vi "H2O_DIAL_NCAR_4CH_v4.06.vi"() -> ()   [LabVIEW 2012]
uses:
  C:/Users/H2ODial/Desktop/Shared Telescope WV DIAL Code/Libraries and VIs/PowerMeterCommands.dll
  Libraries and VIs/PowerMeterCommands.dll
  <vilib>/DAQmx/write.llb/DAQmx Write (Digital 1D Bool NChan 1Samp 1Line).vi
  <vilib>/DAQmx/miscellaneous.llb/DAQmx Fill In Error Info.vi
  <vilib>/Analysis/baseanly.llb/Mean (DBL).vi
  AMCS_Data.vi
  Libraries and VIs/Scalar_Data.vi
  <vilib>/Analysis/NI_AALBase.lvlib
  Libraries and VIs/Scalar_Data_2.vi
  Libraries and VIs/Scalar_Data_4.vi
  Libraries and VIs/Scalar_Data_3.vi
  Libraries and VIs/CLDevIFace.dll
panel:
  out "AMCS_Profile":i32=8
  out "FileHour":i32=17
  out "L_Count":i32=23
  out "sigma_off_total":dbl[](array[numeric])=[5.235525125067343e-25, 5.206358319245337e-25, 5.177318750524933e-25, 5.148406424862825e-25, 5.119621341127451e-25, 5.090963491196627e-25, 5.062432860011865e-25, 5.034029425635027e-25, 5.005753159352157e-25, 4.977604025706667e-25, 4.949581982592347e-25, 4.921686981325722e-25, 4.893918966711095e-25, 4.866277877122191e-25, 4.8387636445644285e-25, 4.811376194764721e-25, 4.784115447230487e-25, 4.756981315339233e-25, 4.729973706394386e-25, 4.703092521721628e-25, 4.6763376567211625e-25, 4.6497090009594435e-25, 4.623206438225019e-25, 4.596829846622293e-25, 4.57057909862005e-25, 4.544454061150213e-25, 4.518454595652437e-25, 4.492580558158126e-25, 4.4668317993693425e-25, 4.441208164702635e-25, 4.41570949437918e-25, 4.390335623482575e-25, 4.365086382028137e-25, 4.339961595028071e-25, 4.314961082547237e-25, 4.290084659777996e-25, 4.2653321370993085e-25, 4.240703320135042e-25, 4.216198009811418e-25, 4.191816002426457e-25, 4.16755708969195e-25, 4.143421058805604e-25, 4.1194076924960845e-25, 4.095516769084665e-25, 4.0717480625238245e-25, 4.0481013424706545e-25, 4.0245763743206737e-25, 4.001172919260011e-25, 3.977890734322512e-25, 3.9547295724256756e-25, 3.931689182419048e-25, 3.908769309139365e-25, 3.8859696934393876e-25, 3.863290072236815e-25, 3.840730178557474e-25, 3.8182897415734565e-25, 3.7959684866403156e-25, 3.773766135338825e-25, 3.7516824055099053e-25, 3.729717011286995e-25, 3.707869663137923e-25, 3.686140067893342e-25, 3.664527928779591e-25, 3.643032945453827e-25, 3.621654814033011e-25, 3.600393227122229e-25, 3.579247873843723e-25, 3.5582184398664743e-25, 3.5373046074361216e-25, 3.5165060553938904e-25, 3.4958224592064764e-25, 3.475253490990589e-25, 3.454798819536632e-25, 3.4344581103303625e-25, 3.414231025576395e-25, 3.394117224218377e-25, 3.37411636196096e-25, 3.3542280912885406e-25, 3.3344520614845767e-25, 3.3147879186525413e-25, 3.295235305730259e-25, 3.275793862509532e-25, 3.2564632256504646e-25, 3.237243028702917e-25, 3.2181329021119735e-25, 3.1991324732434905e-25, 3.180241366390581e-25, 3.161459202790299e-25, 3.142785600633377e-25, 3.1242201750825597e-25, 3.1057625382770893e-25, 3.0874122993477767e-25, 3.0691690644282785e-25, 3.051032436660927e-25, 3.0330020162078266e-25, 3.0150774002602592e-25, 2.997258183045521e-25, 2.979543955833093e-25, 2.961934306943937e-25, 2.944428821752431e-25, 2.9270270826932477e-25, 2.909728669267514e-25, 2.8925331580414936e-25, 2.875440122654977e-25, 2.8584491338173137e-25, 2.841559759313169e-25, 2.8247715639976386e-25, 2.80808410980223e-25, 2.791496955724979e-25, 2.775009657833479e-25, 2.7586217692567447e-25, 2.742332840183121e-25, 2.7261424178518227e-25, 2.710050046547509e-25, 2.6940552675881075e-25, 2.6781576193155516e-25, 2.6623566370876434e-25, 2.646651853260364e-25, 2.6310427971768174e-25, 2.615528995144771e-25, 2.600109970428841e-25, 2.5847852432207883e-25, 2.569554330624564e-25, 2.554416746633416e-25, 2.5393720020962457e-25, 2.5244196047033826e-25, 2.5095590589459477e-25, 2.4947898660936654e-25, 2.480111524155541e-25, 2.4655235278440513e-25, 2.451025368544176e-25, 2.436616534266772e-25, 2.422296509605852e-25, 2.408064775697375e-25, 2.3939208101763006e-25, 2.3798640871112015e-25, 2.365894076971971e-25, 2.352010246556833e-25, 2.3382120589521406e-25, 2.324498973455175e-25, 2.3108704455300754e-25, 2.2973259267270024e-25, 2.283864864626908e-25, 2.270486702764721e-25, 2.257190880557015e-25, 2.2439768332388837e-25, 2.2308439917739663e-25, 2.2177917827749597e-25, 2.20481962844103e-25, 2.19192694645104e-25, 2.179113149897461e-25, 2.166377647190967e-25, 2.153719841983278e-25, 2.1411391330535246e-25, 2.1286349142540036e-25, 2.1162065743868337e-25, 2.103853497130775e-25, 2.091575060946101e-25, 2.079370638983031e-25, 2.0672395989815037e-25, 2.0551813031976677e-25, 2.0431951082869756e-25, 2.0312803652523447e-25, 2.019436419319984e-25, 2.0076626098781596e-25, 1.9959582703908636e-25, 1.9843227283026113e-25, 1.9727553050009988e-25, 1.9612553156963306e-25, 1.9498220693936616e-25, 1.9384548688025462e-25, 1.9271530103114487e-25, 1.915915783921294e-25, 1.9047424731896738e-25, 1.8936323552292957e-25, 1.8825847006561212e-25, 1.8715987735714719e-25, 1.8606738315918164e-25, 1.8498091257941087e-25, 1.8390039007904753e-25, 1.8282573946936752e-25, 1.8175688392200846e-25, 1.80693745969556e-25, 1.7963624751388698e-25, 1.7858430983630522e-25, 1.7753785360393623e-25, 1.7649679888396773e-25, 1.7546106515613228e-25, 1.7443057132789558e-25, 1.7340523575155863e-25, 1.723849762422857e-25, 1.7136971010131167e-25, 1.7035935413825008e-25, 1.6935382469544605e-25, 1.6835303767796407e-25, 1.6735690858143057e-25, 1.6636535252563445e-25, 1.653782842907513e-25, 1.643956183497921e-25, 1.6341726891478545e-25, 1.624431499756322e-25, 1.6147317534796005e-25, 1.6050725871551994e-25, 1.5954531368896971e-25, 1.585872538492723e-25, 1.576329928151117e-25, 1.566824442883223e-25, 1.5573552212546758e-25, 1.5479214039898043e-25, 1.5385221346219397e-25, 1.5291565602013113e-25, 1.519823831962039e-25, 1.5105231061650234e-25, 1.5012535447460145e-25, 1.49201431624485e-25, 1.482804596459418e-25, 1.4736235693849326e-25, 1.46447042805166e-25, 1.455344375360034e-25, 1.4462446250285657e-25, 1.4371704024629248e-25, 1.4281209456557682e-25, 1.4190955061389853e-25, 1.410093350012645e-25, 1.4011137586880333e-25, 1.3921560301221658e-25, 1.3832194795253431e-25, 1.3743034404767374e-25, 1.3654072658699072e-25, 1.3565303288298996e-25, 1.3476720236918642e-25, 1.3388317669734332e-25, 1.3300089982893968e-25, 1.3212031812258562e-25, 1.3124138043688156e-25, 1.3036403820696332e-25, 1.2948824553577423e-25, 1.2861395928315612e-25, 1.2774113913410786e-25, 1.2686974768684636e-25, 1.2599975053009544e-25, 1.2513111630057894e-25, 1.2426381676023619e-25, 1.2339782685325752e-25, 1.2253312476934588e-25, 1.2166969199403071e-25, 1.2080751335374065e-25, 1.1994657705541538e-25, 1.1908687474046665e-25, 1.182284014933639e-25, 1.1737115587808914e-25, 1.1651513996305814e-25, 1.1566035931942852e-25, 1.1480682304187532e-25, 1.1395454373665928e-25, 1.1310353751750977e-25, 1.1225382399779688e-25, 1.1140542626706877e-25, 1.1055837085176348e-25, 1.097126877076807e-25, 1.0886841014622313e-25, 1.0802557481625692e-25, 1.07184221622742e-25, 1.0634439369229237e-25, 1.0550613727868173e-25, 1.0466950171251473e-25, 1.038345393031225e-25, 1.0300130526116006e-25, 1.0216985760646603e-25, 1.0134025706453978e-25, 1.0051256696943142e-25, 9.968685315566847e-26, 9.886318383691271e-26, 9.804162950309608e-26, 9.722226278487634e-26, 9.640515833439737e-26, 9.559039270504641e-26]
  out "sigma_on_total":dbl[](array[numeric])=[2.3995833041051826e-23, 2.3922427806028756e-23, 2.384791688746997e-23, 2.3772317103212935e-23, 2.3695645459223834e-23, 2.3617919143098038e-23, 2.353915551299477e-23, 2.3459372086545772e-23, 2.3378586534805352e-23, 2.3296816668418693e-23, 2.3214080430222583e-23, 2.3130395885585187e-23, 2.3045781211857275e-23, 2.2960254689709635e-23, 2.2873834692216713e-23, 2.2786539677232958e-23, 2.26983881761429e-23, 2.2609398786386177e-23, 2.2519590159903235e-23, 2.2428980996764618e-23, 2.233759003334336e-23, 2.2245436035687533e-23, 2.215253778837344e-23, 2.2058914088573995e-23, 2.1964583734229998e-23, 2.1869565519300118e-23, 2.1773878221738038e-23, 2.1677540597169405e-23, 2.1580571372247846e-23, 2.1482989233079665e-23, 2.1384812820738464e-23, 2.1286060722317668e-23, 2.11867514639952e-23, 2.108690350380322e-23, 2.0986535223192663e-23, 2.0885664921990106e-23, 2.078431081122936e-23, 2.068249100616584e-23, 2.0580223519476976e-23, 2.0477526256926665e-23, 2.037441700865306e-23, 2.0270913446113544e-23, 2.0167033114661947e-23, 2.0062793429495973e-23, 1.9958211667723764e-23, 1.985330496739564e-23, 1.9748090319499057e-23, 1.9642584563764407e-23, 1.9536804385991807e-23, 1.9430766311537824e-23, 1.9324486701686134e-23, 1.9217981751967428e-23, 1.9111267485338587e-23, 1.9004359749995074e-23, 1.889727421646792e-23, 1.8790026374021327e-23, 1.8682631527238793e-23, 1.8575104794097395e-23, 1.84674611029044e-23, 1.835971518898627e-23, 1.8251881594141955e-23, 1.814397466323634e-23, 1.803600854226578e-23, 1.7927997177436358e-23, 1.781995431311586e-23, 1.7711893489953737e-23, 1.7603828043585478e-23, 1.7495771103906582e-23, 1.7387735594900776e-23, 1.7279734231695694e-23, 1.7171779521110194e-23, 1.7063883761078407e-23, 1.6956059040208986e-23, 1.6848317237070065e-23, 1.6740670020423286e-23, 1.663312884876634e-23, 1.6525704970810114e-23, 1.6418409425264909e-23, 1.6311253041149504e-23, 1.6204246439001306e-23, 1.6097400030205636e-23, 1.5990724018419113e-23, 1.5884228399513838e-23, 1.577792296435066e-23, 1.5671817296197546e-23, 1.5565920775619874e-23, 1.5460242578862832e-23, 1.535479168018885e-23, 1.5249576851998408e-23, 1.514460666843388e-23, 1.5039889504141115e-23, 1.4935433537260487e-23, 1.4831246751329234e-23, 1.472733693540472e-23, 1.4623711686480822e-23, 1.4520378411573963e-23, 1.4417344329131002e-23, 1.431461647050052e-23, 1.4212201682885124e-23, 1.4110106629829185e-23, 1.4008337793905047e-23, 1.3906901479412008e-23, 1.3805803812661607e-23, 1.3705050746147406e-23, 1.360464805856419e-23, 1.3504601358671784e-23, 1.3404916085744038e-23, 1.33055975141312e-23, 1.3206650752755123e-23, 1.3108080749361715e-23, 1.300989229142433e-23, 1.2912090009400432e-23, 1.2814678378339959e-23, 1.2717661720819296e-23, 1.2621044208258517e-23, 1.2524829863555887e-23, 1.2429022564345148e-23, 1.2333626044024168e-23, 1.2238643895015358e-23, 1.2144079569516218e-23, 1.2049936384300202e-23, 1.1956217520538888e-23, 1.1862926027653837e-23, 1.1770064825596866e-23, 1.1677636705336423e-23, 1.1585644333848872e-23, 1.1494090253993612e-23, 1.140297688856002e-23, 1.1312306541333314e-23, 1.1222081399347362e-23, 1.1132303536262725e-23, 1.1042974913417118e-23, 1.095409738203383e-23, 1.0865672685970165e-23, 1.077770246442273e-23, 1.069018825184856e-23, 1.0603131482864411e-23, 1.0516533491872498e-23, 1.0430395517331488e-23, 1.0344718701655819e-23, 1.0259504095410726e-23, 1.0174752657463625e-23, 1.0090465258313015e-23, 1.0006642681274029e-23, 9.92328562444393e-24, 9.840394703656403e-24, 9.757970453103036e-24, 9.676013327237633e-24, 9.594523704137527e-24, 9.513501885337853e-24, 9.432948099139377e-24, 9.352862501650117e-24, 9.273245179271553e-24, 9.194096148754277e-24, 9.115415361305784e-24, 9.037202702127212e-24, 8.95945799326533e-24, 8.882180995005424e-24, 8.805371407477425e-24, 8.729028871786063e-24, 8.653152972477945e-24, 8.577743237723576e-24, 8.502799142614571e-24, 8.428320108863437e-24, 8.354305507372407e-24, 8.280754659437585e-24, 8.207666837515396e-24, 8.135041268097952e-24, 8.062877131154292e-24, 7.99117356294852e-24, 7.919929656301442e-24, 7.84914446290975e-24, 7.778816993979177e-24, 7.708946221065343e-24, 7.639531078293294e-24, 7.570570462739891e-24, 7.50206323561057e-24, 7.434008224352779e-24, 7.366404222220212e-24, 7.299249990914871e-24, 7.232544260133964e-24, 7.166285730139122e-24, 7.100473071653504e-24, 7.035104927252298e-24, 6.970179912711283e-24, 6.905696617243793e-24, 6.841653604993835e-24, 6.778049415778176e-24, 6.71488256599146e-24, 6.652151549491076e-24, 6.5898548382920406e-24, 6.527990883757523e-24, 6.466558117249894e-24, 6.4055549507723266e-24, 6.344979778092631e-24, 6.28483097518053e-24, 6.225106901127807e-24, 6.165805899041039e-24, 6.106926296119407e-24, 6.048466405156796e-24, 5.9904245247443424e-24, 5.932798940248885e-24, 5.875587923847452e-24, 5.81878973608226e-24, 5.762402625414115e-24, 5.7064248300296764e-24, 5.6508545770856186e-24, 5.595690084324867e-24, 5.540929560331407e-24, 5.4865712049292154e-24, 5.432613209855631e-24, 5.379053758857358e-24, 5.325891029033336e-24, 5.273123190347269e-24, 5.220748407202883e-24, 5.1687648376764325e-24, 5.117170634787307e-24, 5.065963946793787e-24, 5.015142917355626e-24, 4.964705686339599e-24, 4.914650389956907e-24, 4.864975161029941e-24, 4.81567812950341e-24, 4.766757423304431e-24, 4.718211167461553e-24, 4.670037486052705e-24, 4.622234501071692e-24, 4.574800333610437e-24, 4.5277331040472795e-24, 4.4810309321178136e-24, 4.4346919373328924e-24, 4.38871423937983e-24, 4.3430959582840964e-24, 4.297835214458712e-24, 4.252930129523995e-24, 4.208378826002288e-24, 4.164179427788139e-24, 4.120330060596267e-24, 4.0768288516550796e-24, 4.033673930358468e-24, 3.990863428575472e-24, 3.9483954803378585e-24, 3.9062682224559106e-24, 3.8644797945055325e-24, 3.823028339213923e-24, 3.781912002534402e-24, 3.741128933721167e-24, 3.700677285403917e-24, 3.660555214319274e-24, 3.620760880699127e-24, 3.581292448804293e-24, 3.5421480872458e-24, 3.5033259686601366e-24, 3.4648242702967565e-24, 3.4266411737802344e-24, 3.3887748653248774e-24, 3.35122353602395e-24, 3.313985381867669e-24, 3.2770586035106233e-24, 3.2404414071352855e-24, 3.2041320036199322e-24, 3.168128609466342e-24, 3.1324294461445785e-24, 3.097032740909227e-24, 3.061936726152549e-24, 3.0271396401184125e-24, 2.9926397264979493e-24, 2.958435234734132e-24, 2.9245244200823504e-24, 2.8909055435197247e-24, 2.857576871953275e-24, 2.8245366782699725e-24, 2.7917832411696796e-24, 2.7593148455736252e-24, 2.727129782308357e-24, 2.6952263482932426e-24, 2.663602846782851e-24]
  out "background start":u32=269
  in  "Tab Control 2":enum32{"WV ND far", "WV ND near"}(tab)
  out "Water Vapor Number Density":dbl[][](graph)=[[-1.2429232877484484, -0.1516675083101968, -0.2538905255591858, -0.8248790705144008, -0.7242099736682136, -0.00381566942216356, 0.5865003613322888, 0.8338027871213243, 0.9701605815337504, 1.1834523029548778, 1.5190287098751127, 1.7810431574320749, 1.6746765343626566, 1.1151725227331368, 0.46655235793116506, 0.35715468660627175, 0.6669999198229103, 0.6229583187384804, 0.5589044475896486, 0.7015386580818149, 0.4798277530250588, 0.5321622767939538, 0.7626570360936702, 0.548610948648949, 0.9084936586508549, 1.2026792009723286, 0.774704699408754, 0.5215060631479779, 0.12261891062905873, 0.21928947886161568, 0.8338105270444128, 0.7207357046057596, 0.7010869622309128, 1.3141939911674185, 0.9797233881152331, 0.17444693844264145, 0.8196905370743147, 1.2982930105898909, 0.11109624339884688, -0.43162778210005126, 0.5989210399599628, 0.8290997131095186, 0.9085277187984653, 1.1666295347768159, 1.4953864166373505, 0.973830244036953, 0.40024763155462806, 0.40566207310085767, 0.12859842661309212, 0.816329506196804, 1.6877091211861164, 1.4740247437794118, 0.5494960806690096, 0.14364505636130315, 1.6910867165083499, 2.541349269410972, 3.0215147517757615, 5.116023264360957, 11.66361642135062, 15.732511596518307, 11.746439379020979, 10.179584454030591, 9.832529406708609, 8.268647831389469, 4.724342168222102, -5.092206912585782, -13.3625201348692, -20.76218607865762, -31.481285721313007, -38.11141827571821, -31.134574912835927, -23.05395421124333, -18.75920646807871, -11.6291784332, -9.182440744289961, 3.6065364004744884, 14.28272592509906, 16.011915781887442, 21.469311288754138, 22.06574013828088, 12.21267680703055, 7.045281295181791, 5.126441440726531, 2.1140699610393394, 4.549659394917577, 5.4053975728869545, -1.494856115972021, -1.1471850648222977, -2.2964282267520684, -1.701978840115399, 6.926942778338519, -5.157508026215396, -16.63199538963445, -9.965627988382359, -9.996745428358686, -11.837454532000542, -7.791885667567633, -8.680656157447176, -8.91275723505151, -1.6980976668310848, -2.133416024855749, 6.9027910551985565, 15.630215820196536, 9.119408516902418, 13.419777247258404, 3.714772754413472, -1.0207358839785408, 1.9570108859042183, 8.45768550919551, 5.500832494929015, 9.619107112547066, 3.5429906655082815, 2.281420809371128, 3.3348498361329115, 13.33869517507839, 20.282683395031995, 12.958395546058279, 12.790251903025284, 5.239171426669377, 5.18576865128037, -7.793357814133322, -4.368293566880555, -3.168338430754624, -3.568868023379041, -19.349826708428175, -18.20847151281235, -6.272910319204182, -5.810405292731198, 0.03778017829370816, 1.6447693871034739, 12.138812274569242, 22.264002949155152, 20.98736700005724, 5.225366734954423, -4.2130058766847345, -5.530836082222857, -7.678583545699047, 2.8238125624467885, 4.404424187372618, -16.837237405438508, -25.11428016723591, -32.56648715841542, -51.93781123610291, -12.449234368136176, -7.120712329696384, -7.810751630429527, -5.682295948947324, -14.881668117301965, -17.89571509714611, 21.5597299249097, 14.887365183365386, 9.094029084786875, 39.765998068462736, 26.698821470330174, 5.3888067881035235, 36.31266939640943, 23.52473002015805, 7.885320353358003, 4.491673034757693, -25.66484118463619, -24.784846332156523, -11.314522471658744, -8.629722713276472, -36.47960588329874, 3.344643837569838, -43.4685580824685, -21.017479049621816, -13.573236011339208, 1.4056605605320718, 20.621744510192077, 48.534446642723786, 18.043662576249712, 18.729984852689935, 15.453816513065464, -16.562572588412568, -1.75727853159035, 12.077447417423167, 23.28859626581528, 8.189331760622546, -10.325523115047803, -24.985943747309573, 11.02611193863362, -21.194886596636273, -3.3737336795583666, 12.356163073717218, 19.49913906422601, -31.903517194256743, -28.34741638064177, -22.84649773688388, -3.7322150184329868, -7.133598473140854, -30.506891256676347, 0.8094334644236778, -10.185875717445333, -1.7805612059650464, -18.920780567052645, 18.561020494796015, 32.740090001051776, -10.431965025082278, 24.148735007779216, -12.811558818079975, 22.77751095878245, 3.073515709862989, -1.5964031788087782, 23.237423290854288, -10.171927114726072, -18.071924640995153, -22.573720000403977, 31.51068338334455, -25.15388772107271, -10.403629581588998, -23.273123302299926, -0.7696347470225127, 28.138111524189863, -53.130668832773836, 19.25820068507475, 30.433478138971022, 4.601226158871911, -7.687709637981916, 26.504732966928117, -6.453108031183767, 12.133560044433468, -17.91335412457681, -27.611164781409965, 58.267542043909756, 27.655747672019785, 10.074228863403778, -15.797465265403272, 29.104671664483025, -20.527102926569924, 71.93119794505054, 8.975498249493553, -3.3375393334362444, 25.152309034601856, -9.70197245913663, -28.78587032628703, -37.26876049881305, -21.358169118247066, -42.25654771519554, 38.05236561426804, -21.06199519179915, -19.681897042577624, -33.54178592739098, -8.38025346936163, -9.769431139416938, 11.584675554539887, 6.052684205738731, 15.000220216910806, -37.12617526141696, -19.779582424384554, 7.072374690381783, 9.593917717650474, 9.722908351927563, -19.755356323145175, 1.5520809859448423, 32.36319254600239, 31.348864192718274, -34.65191626742631, 18.898751794149703, -13.173451913530773, -79.37971946570717, -82.26941833977881, 51.361564922853184, 37.72821751239603, 23.664211401877278, -159.38500039414865, 63.63015044438198, 87.46258784324492, 124.20770000486162, 110.10692816340169, 58.297939579874345, 90.76767995026964, -0.5951627932311193, -15.350600261615488, -23.944134589509243, 130.0552581066162, 0.0, 0.0, 0.0, 0.0]]
  out "Water Vapor Number Density 2":dbl[][](graph)=[[nan, nan, nan, nan, nan, nan, nan, nan, nan, nan, nan, nan, nan, nan, nan, nan, nan, nan, nan, nan, nan, nan, nan, nan, nan, nan, nan, nan, nan, nan, nan, nan, nan, nan, nan, nan, nan, nan, nan, nan, nan, nan, nan, nan, nan, nan, nan, nan, nan, nan, nan, nan, nan, nan, nan, nan, nan, nan, nan, nan, nan, nan, nan, nan, nan, nan, nan, nan, nan, nan, nan, nan, nan, nan, nan, nan, nan, nan, nan, nan, nan, nan, nan, nan, nan, nan, nan, nan, nan, nan, nan, nan, nan, nan, nan, nan, nan, nan, nan, nan, nan, nan, nan, nan, nan, nan, nan, nan, nan, nan, nan, nan, nan, nan, nan, nan, nan, nan, nan, nan, nan, nan, nan, nan, nan, nan, nan, nan, nan, nan, nan, nan, nan, nan, nan, nan, nan, nan, nan, nan, nan, nan, nan, nan, nan, nan, nan, nan, nan, nan, nan, nan, nan, nan, nan, nan, nan, nan, nan, nan, nan, nan, nan, nan, nan, nan, nan, nan, nan, nan, nan, nan, nan, nan, nan, nan, nan, nan, nan, nan, nan, nan, nan, nan, nan, nan, nan, nan, nan, nan, nan, nan, nan, nan, nan, nan, nan, nan, nan, nan, nan, nan, nan, nan, nan, nan, nan, nan, nan, nan, nan, nan, nan, nan, nan, nan, nan, nan, nan, nan, nan, nan, nan, nan, nan, nan, nan, nan, nan, nan, nan, nan, nan, nan, nan, nan, nan, nan, nan, nan, nan, nan, nan, nan, nan, nan, nan, nan, nan, nan, nan, nan, nan, nan, nan, nan, nan, nan, nan, nan, nan, nan, nan, nan, nan, nan, nan, nan, nan, nan, nan, nan, nan, nan, nan, nan, 0.0, 0.0, 0.0, 0.0]] caption="Water Vapor Number Density"
  out "RingBuffer offline near":dbl[][](array[numeric])
  out "RingBuffer aerosol near":dbl[][](array[numeric])
  in  "?":T1(tab)=enum."Raw Counts far"
  out "NRB":dbl[][](graph)=[[nan, nan, nan, nan, nan, nan, nan, nan, nan, nan, nan, nan, nan, nan, nan, nan, nan, nan, nan, nan, nan, nan, nan, nan, nan, nan, nan, nan, nan, nan, nan, nan, nan, nan, nan, nan, nan, nan, nan, nan, nan, nan, nan, nan, nan, nan, nan, nan, nan, nan, nan, nan, nan, nan, nan, nan, nan, nan, nan, nan, nan, nan, nan, nan, nan, nan, nan, nan, nan, nan, nan, nan, nan, nan, nan, nan, nan, nan, nan, nan, nan, nan, nan, nan, nan, nan, nan, nan, nan, nan, nan, nan, nan, nan, nan, nan, nan, nan, nan, nan, nan, nan, nan, nan, nan, nan, nan, nan, nan, nan, nan, nan, nan, nan, nan, nan, nan, nan, nan, nan, nan, nan, nan, nan, nan, nan, nan, nan, nan, nan, nan, nan, nan, nan, nan, nan, nan, nan, nan, nan, nan, nan, nan, nan, nan, nan, nan, nan, nan, nan, nan, nan, nan, nan, nan, nan, nan, nan, nan, nan, nan, nan, nan, nan, nan, nan, nan, nan, nan, nan, nan, nan, nan, nan, nan, nan, nan, nan, nan, nan, nan, nan, nan, nan, nan, nan, nan, nan, nan, nan, nan, nan, nan, nan, nan, nan, nan, nan, nan, nan, nan, nan, nan, nan, nan, nan, nan, nan, nan, nan, nan, nan, nan, nan, nan, nan, nan, nan, nan, nan, nan, nan, nan, nan, nan, nan, nan, nan, nan, nan, nan, nan, nan, nan, nan, nan, nan, nan, nan, nan, nan, nan, nan, nan, nan, nan, nan, nan, nan, nan, nan, nan, nan, nan, nan, nan, nan, nan, nan, nan, nan, nan, nan, nan, nan, nan, nan, nan, nan, nan, nan, nan, nan, nan, nan, nan, nan, 0.0, 0.0, 0.0]] caption="Water Vapor Number Density"
  out "NRB 2":dbl[][](graph)=[[nan, nan, nan, nan, nan, nan, nan, nan, nan, nan, nan, nan, nan, nan, nan, nan, nan, nan, nan, nan, nan, nan, nan, nan, nan, nan, nan, nan, nan, nan, nan, nan, nan, nan, nan, nan, nan, nan, nan, nan, nan, nan, nan, nan, nan, nan, nan, nan, nan, nan, nan, nan, nan, nan, nan, nan, nan, nan, nan, nan, nan, nan, nan, nan, nan, nan, nan, nan, nan, nan, nan, nan, nan, nan, nan, nan, nan, nan, nan, nan, nan, nan, nan, nan, nan, nan, nan, nan, nan, nan, nan, nan, nan, nan, nan, nan, nan, nan, nan, nan, nan, nan, nan, nan, nan, nan, nan, nan, nan, nan, nan, nan, nan, nan, nan, nan, nan, nan, nan, nan, nan, nan, nan, nan, nan, nan, nan, nan, nan, nan, nan, nan, nan, nan, nan, nan, nan, nan, nan, nan, nan, nan, nan, nan, nan, nan, nan, nan, nan, nan, nan, nan, nan, nan, nan, nan, nan, nan, nan, nan, nan, nan, nan, nan, nan, nan, nan, nan, nan, nan, nan, nan, nan, nan, nan, nan, nan, nan, nan, nan, nan, nan, nan, nan, nan, nan, nan, nan, nan, nan, nan, nan, nan, nan, nan, nan, nan, nan, nan, nan, nan, nan, nan, nan, nan, nan, nan, nan, nan, nan, nan, nan, nan, nan, nan, nan, nan, nan, nan, nan, nan, nan, nan, nan, nan, nan, nan, nan, nan, nan, nan, nan, nan, nan, nan, nan, nan, nan, nan, nan, nan, nan, nan, nan, nan, nan, nan, nan, nan, nan, nan, nan, nan, nan, nan, nan, nan, nan, nan, nan, nan, nan, nan, nan, nan, nan, nan, nan, nan, nan, nan, nan, nan, nan, nan, nan, nan, 0.0, 0.0, 0.0]] caption="Water Vapor Number Density"
  out "raw counts":dbl[][](graph) caption="Water Vapor Number Density"
  out "raw counts near":dbl[][](graph) caption="Water Vapor Number Density"
  out "Aerosol Smoothed 2":dbl[](array[numeric])
  out "Off-Line Smoothed 2":dbl[](array[numeric])
  out "Off-Line Bin Readings 2":dbl[](array[numeric])
  out "On-Line Smoothed 2":dbl[](array[numeric])
  out "On-Line Bin Readings 2":dbl[](array[numeric])
  in  "stop":bool
  in  "Reset Average":bool=TRUE
  in  "Save Data?":bool=TRUE
  in  "Collect Data?":bool=TRUE
  in  "ILX Address":i32=6 min=0 step=1
  in  "Lambda On DBR Current":dbl=170.37999999999937
  in  "Lambda Off DBR Current":dbl=172.63
  in  "Tab Control":T2(tab)=enum."g/m^3"
  out "Water Vapor Number Density  2":cluster{"Y":dbl[], "Y":dbl[]}[](graph)=[{"Y"=array[276 elements], "Y"=array[280 elements]}, {"Y"=[nan, nan, nan, nan, nan, nan, nan, nan, nan, nan, nan, nan, nan, nan, nan, nan, nan, nan, nan, nan, nan, nan, nan, nan, nan, nan, nan, nan, nan, nan, nan, nan, nan, nan, nan, nan, nan, nan, nan, nan, nan, nan, nan, nan, nan, nan, nan, nan, nan, nan, nan, nan, nan, nan, nan, nan, nan, nan, nan, nan, nan, nan, nan, nan, nan, nan, nan, nan, nan, nan, nan, nan, nan, nan, nan, nan, nan, nan, nan, nan, nan, nan, nan, nan, nan, nan, nan, nan, nan, nan, nan, nan, nan, nan, nan, nan, nan, nan, nan, nan, nan, nan, nan, nan, nan, nan, nan, nan, nan, nan, nan, nan, nan, nan, nan, nan, nan, nan, nan, nan, nan, nan, nan, nan, nan, nan, nan, nan, nan, nan, nan, nan, nan, nan, nan, nan, nan, nan, nan, nan, nan, nan, nan, nan, nan, nan, nan, nan, nan, nan, nan, nan, nan, nan, nan, nan, nan, nan, nan, nan, nan, nan, nan, nan, nan, nan, nan, nan, nan, nan, nan, nan, nan, nan, nan, nan, nan, nan, nan, nan, nan, nan, nan, nan, nan, nan, nan, nan, nan, nan, nan, nan, nan, nan, nan, nan, nan, nan, nan, nan, nan, nan, nan, nan, nan, nan, nan, nan, nan, nan, nan, nan, nan, nan, nan, nan, nan, nan, nan, nan, nan, nan, nan, nan, nan, nan, nan, nan, nan, nan, nan, nan, nan, nan, nan, nan, nan, nan, nan, nan, nan, nan, nan, nan, nan, nan, nan, nan, nan, nan, nan, nan, nan, nan, nan, nan, nan, nan, nan, nan, nan, nan, nan, nan, nan, nan, nan, nan, nan, nan, nan, nan, nan, nan, nan, nan], "Y"=array[280 elements]}]
  out "Absolute Humidity":cluster{"Y":dbl[], "Y":dbl[]}[](graph)=[{"Y"=array[276 elements], "Y"=array[280 elements]}, {"Y"=[nan, nan, nan, nan, nan, nan, nan, nan, nan, nan, nan, nan, nan, nan, nan, nan, nan, nan, nan, nan, nan, nan, nan, nan, nan, nan, nan, nan, nan, nan, nan, nan, nan, nan, nan, nan, nan, nan, nan, nan, nan, nan, nan, nan, nan, nan, nan, nan, nan, nan, nan, nan, nan, nan, nan, nan, nan, nan, nan, nan, nan, nan, nan, nan, nan, nan, nan, nan, nan, nan, nan, nan, nan, nan, nan, nan, nan, nan, nan, nan, nan, nan, nan, nan, nan, nan, nan, nan, nan, nan, nan, nan, nan, nan, nan, nan, nan, nan, nan, nan, nan, nan, nan, nan, nan, nan, nan, nan, nan, nan, nan, nan, nan, nan, nan, nan, nan, nan, nan, nan, nan, nan, nan, nan, nan, nan, nan, nan, nan, nan, nan, nan, nan, nan, nan, nan, nan, nan, nan, nan, nan, nan, nan, nan, nan, nan, nan, nan, nan, nan, nan, nan, nan, nan, nan, nan, nan, nan, nan, nan, nan, nan, nan, nan, nan, nan, nan, nan, nan, nan, nan, nan, nan, nan, nan, nan, nan, nan, nan, nan, nan, nan, nan, nan, nan, nan, nan, nan, nan, nan, nan, nan, nan, nan, nan, nan, nan, nan, nan, nan, nan, nan, nan, nan, nan, nan, nan, nan, nan, nan, nan, nan, nan, nan, nan, nan, nan, nan, nan, nan, nan, nan, nan, nan, nan, nan, nan, nan, nan, nan, nan, nan, nan, nan, nan, nan, nan, nan, nan, nan, nan, nan, nan, nan, nan, nan, nan, nan, nan, nan, nan, nan, nan, nan, nan, nan, nan, nan, nan, nan, nan, nan, nan, nan, nan, nan, nan, nan, nan, nan, nan, nan, nan, nan, nan, nan], "Y"=array[280 elements]}]
  out "NRB plot":cluster{"Y":dbl[], "Y":dbl[]}[](graph)=[{"Y"=[nan, nan, nan, nan, nan, nan, nan, nan, nan, nan, nan, nan, nan, nan, nan, nan, nan, nan, nan, nan, nan, nan, nan, nan, nan, nan, nan, nan, nan, nan, nan, nan, nan, nan, nan, nan, nan, nan, nan, nan, nan, nan, nan, nan, nan, nan, nan, nan, nan, nan, nan, nan, nan, nan, nan, nan, nan, nan, nan, nan, nan, nan, nan, nan, nan, nan, nan, nan, nan, nan, nan, nan, nan, nan, nan, nan, nan, nan, nan, nan, nan, nan, nan, nan, nan, nan, nan, nan, nan, nan, nan, nan, nan, nan, nan, nan, nan, nan, nan, nan, nan, nan, nan, nan, nan, nan, nan, nan, nan, nan, nan, nan, nan, nan, nan, nan, nan, nan, nan, nan, nan, nan, nan, nan, nan, nan, nan, nan, nan, nan, nan, nan, nan, nan, nan, nan, nan, nan, nan, nan, nan, nan, nan, nan, nan, nan, nan, nan, nan, nan, nan, nan, nan, nan, nan, nan, nan, nan, nan, nan, nan, nan, nan, nan, nan, nan, nan, nan, nan, nan, nan, nan, nan, nan, nan, nan, nan, nan, nan, nan, nan, nan, nan, nan, nan, nan, nan, nan, nan, nan, nan, nan, nan, nan, nan, nan, nan, nan, nan, nan, nan, nan, nan, nan, nan, nan, nan, nan, nan, nan, nan, nan, nan, nan, nan, nan, nan, nan, nan, nan, nan, nan, nan, nan, nan, nan, nan, nan, nan, nan, nan, nan, nan, nan, nan, nan, nan, nan, nan, nan, nan, nan, nan, nan, nan, nan, nan, nan, nan, nan, nan, nan, nan, nan, nan, nan, nan, nan, nan, nan, nan, nan, nan, nan, nan, nan, nan, nan, nan, nan, nan, nan, nan, nan, nan, nan, nan], "Y"=[0.075, 0.15, 0.22499999999999998, 0.3, 0.375, 0.45, 0.5249999999999999, 0.6, 0.6749999999999999, 0.7499999999999999, 0.825, 0.8999999999999999, 0.9749999999999999, 1.05, 1.125, 1.2, 1.275, 1.3499999999999999, 1.4249999999999998, 1.5, 1.575, 1.65, 1.7249999999999999, 1.7999999999999998, 1.8749999999999998, 1.95, 2.025, 2.1, 2.1750000000000003, 2.25, 2.325, 2.4, 2.475, 2.5500000000000003, 2.625, 2.7, 2.775, 2.85, 2.9250000000000003, 3.0, 3.075, 3.15, 3.225, 3.3000000000000003, 3.375, 3.45, 3.525, 3.6, 3.675, 3.75, 3.825, 3.9, 3.975, 4.05, 4.125, 4.2, 4.275, 4.35, 4.425, 4.5, 4.575, 4.65, 4.725, 4.8, 4.875, 4.95, 5.025, 5.1, 5.175, 5.25, 5.325, 5.4, 5.475, 5.55, 5.625, 5.7, 5.775, 5.85, 5.925, 6.0, 6.075, 6.15, 6.225, 6.3, 6.375, 6.45, 6.525, 6.6, 6.675, 6.75, 6.825, 6.9, 6.975, 7.05, 7.125, 7.2, 7.2749999999999995, 7.35, 7.425, 7.5, 7.575, 7.6499999999999995, 7.725, 7.8, 7.875, 7.95, 8.024999999999999, 8.1, 8.174999999999999, 8.249999999999998, 8.325, 8.399999999999999, 8.475, 8.549999999999999, 8.624999999999998, 8.7, 8.774999999999999, 8.85, 8.924999999999999, 8.999999999999998, 9.075, 9.149999999999999, 9.225, 9.299999999999999, 9.374999999999998, 9.45, 9.524999999999999, 9.6, 9.674999999999999, 9.749999999999998, 9.825, 9.899999999999999, 9.975, 10.049999999999999, 10.124999999999998, 10.2, 10.274999999999999, 10.35, 10.424999999999999, 10.499999999999998, 10.575, 10.649999999999999, 10.725, 10.799999999999999, 10.874999999999998, 10.95, 11.024999999999999, 11.1, 11.174999999999999, 11.249999999999998, 11.325, 11.399999999999999, 11.475, 11.549999999999999, 11.624999999999998, 11.7, 11.774999999999999, 11.85, 11.924999999999999, 11.999999999999998, 12.075, 12.149999999999999, 12.225, 12.299999999999999, 12.374999999999998, 12.45, 12.524999999999999, 12.6, 12.674999999999999, 12.749999999999998, 12.825, 12.899999999999999, 12.975, 13.049999999999999, 13.124999999999998, 13.2, 13.274999999999999, 13.35, 13.424999999999999, 13.499999999999998, 13.575, 13.649999999999999, 13.725, 13.799999999999999, 13.874999999999998, 13.95, 14.024999999999999, 14.1, 14.174999999999999, 14.249999999999998, 14.325, 14.399999999999999, 14.474999999999998, 14.549999999999999, 14.624999999999998, 14.7, 14.774999999999999, 14.849999999999998, 14.924999999999999, 14.999999999999998, 15.075, 15.149999999999999, 15.224999999999998, 15.299999999999999, 15.374999999999998, 15.45, 15.524999999999999, 15.599999999999998, 15.674999999999999, 15.749999999999998, 15.825, 15.899999999999999, 15.974999999999998, 16.05, 16.125, 16.2, 16.275, 16.349999999999998, 16.424999999999997, 16.5, 16.575, 16.65, 16.724999999999998, 16.799999999999997, 16.875, 16.95, 17.025, 17.099999999999998, 17.174999999999997, 17.25, 17.325, 17.4, 17.474999999999998, 17.549999999999997, 17.625, 17.7, 17.775, 17.849999999999998, 17.924999999999997, 18.0, 18.075, 18.15, 18.224999999999998, 18.299999999999997, 18.375, 18.45, 18.525, 18.599999999999998, 18.674999999999997, 18.75, 18.825, 18.9, 18.974999999999998, 19.049999999999997, 19.125, 19.2, 19.275, 19.349999999999998, 19.424999999999997, 19.5, 19.575, 19.65, 19.724999999999998, 19.799999999999997, 19.875, 19.95, 20.025, 20.099999999999998, 20.174999999999997, 20.25, 20.325, 20.4, 20.474999999999998, 20.549999999999997, 20.625, 20.7, 20.775, 20.849999999999998, 20.924999999999997, 21.0]}, ...(2 in all)]
  in  "background length":i32=10
  out "Correction":cluster{"Y":dbl[], "Y":dbl[]}[](graph)=[{"Y"=[nan, nan, nan, nan, nan, nan, nan, nan, nan, nan, nan, nan, nan, nan, nan, nan, nan, nan, nan, nan, nan, nan, nan, nan, nan, nan, nan, nan, nan, nan, nan, nan, nan, nan, nan, nan, nan, nan, nan, nan, nan, nan, nan, nan, nan, nan, nan, nan, nan, nan, nan, nan, nan, nan, nan, nan, nan, nan, nan, nan, nan, nan, nan, nan, nan, nan, nan, nan, nan, nan, nan, nan, nan, nan, nan, nan, nan, nan, nan, nan, nan, nan, nan, nan, nan, nan, nan, nan, nan, nan, nan, nan, nan, nan, nan, nan, nan, nan, nan, nan, nan, nan, nan, nan, nan, nan, nan, nan, nan, nan, nan, nan, nan, nan, nan, nan, nan, nan, nan, nan, nan, nan, nan, nan, nan, nan, nan, nan, nan, nan, nan, nan, nan, nan, nan, nan, nan, nan, nan, nan, nan, nan, nan, nan, nan, nan, nan, nan, nan, nan, nan, nan, nan, nan, nan, nan, nan, nan, nan, nan, nan, nan, nan, nan, nan, nan, nan, nan, nan, nan, nan, nan, nan, nan, nan, nan, nan, nan, nan, nan, nan, nan, nan, nan, nan, nan, nan, nan, nan, nan, nan, nan, nan, nan, nan, nan, nan, nan, nan, nan, nan, nan, nan, nan, nan, nan, nan, nan, nan, nan, nan, nan, nan, nan, nan, nan, nan, nan, nan, nan, nan, nan, nan, nan, nan, nan, nan, nan, nan, nan, nan, nan, nan, nan, nan, nan, nan, nan, nan, nan, nan, nan, nan, nan, nan, nan, nan, nan, nan, nan, nan, nan, nan, nan, nan, nan, nan, nan, nan, nan, nan, nan, nan, nan, nan, nan, nan, nan, nan, nan, nan, nan, nan, nan, nan, nan, nan], "Y"=[0.075, 0.15, 0.22499999999999998, 0.3, 0.375, 0.45, 0.5249999999999999, 0.6, 0.6749999999999999, 0.7499999999999999, 0.825, 0.8999999999999999, 0.9749999999999999, 1.05, 1.125, 1.2, 1.275, 1.3499999999999999, 1.4249999999999998, 1.5, 1.575, 1.65, 1.7249999999999999, 1.7999999999999998, 1.8749999999999998, 1.95, 2.025, 2.1, 2.1750000000000003, 2.25, 2.325, 2.4, 2.475, 2.5500000000000003, 2.625, 2.7, 2.775, 2.85, 2.9250000000000003, 3.0, 3.075, 3.15, 3.225, 3.3000000000000003, 3.375, 3.45, 3.525, 3.6, 3.675, 3.75, 3.825, 3.9, 3.975, 4.05, 4.125, 4.2, 4.275, 4.35, 4.425, 4.5, 4.575, 4.65, 4.725, 4.8, 4.875, 4.95, 5.025, 5.1, 5.175, 5.25, 5.325, 5.4, 5.475, 5.55, 5.625, 5.7, 5.775, 5.85, 5.925, 6.0, 6.075, 6.15, 6.225, 6.3, 6.375, 6.45, 6.525, 6.6, 6.675, 6.75, 6.825, 6.9, 6.975, 7.05, 7.125, 7.2, 7.2749999999999995, 7.35, 7.425, 7.5, 7.575, 7.6499999999999995, 7.725, 7.8, 7.875, 7.95, 8.024999999999999, 8.1, 8.174999999999999, 8.249999999999998, 8.325, 8.399999999999999, 8.475, 8.549999999999999, 8.624999999999998, 8.7, 8.774999999999999, 8.85, 8.924999999999999, 8.999999999999998, 9.075, 9.149999999999999, 9.225, 9.299999999999999, 9.374999999999998, 9.45, 9.524999999999999, 9.6, 9.674999999999999, 9.749999999999998, 9.825, 9.899999999999999, 9.975, 10.049999999999999, 10.124999999999998, 10.2, 10.274999999999999, 10.35, 10.424999999999999, 10.499999999999998, 10.575, 10.649999999999999, 10.725, 10.799999999999999, 10.874999999999998, 10.95, 11.024999999999999, 11.1, 11.174999999999999, 11.249999999999998, 11.325, 11.399999999999999, 11.475, 11.549999999999999, 11.624999999999998, 11.7, 11.774999999999999, 11.85, 11.924999999999999, 11.999999999999998, 12.075, 12.149999999999999, 12.225, 12.299999999999999, 12.374999999999998, 12.45, 12.524999999999999, 12.6, 12.674999999999999, 12.749999999999998, 12.825, 12.899999999999999, 12.975, 13.049999999999999, 13.124999999999998, 13.2, 13.274999999999999, 13.35, 13.424999999999999, 13.499999999999998, 13.575, 13.649999999999999, 13.725, 13.799999999999999, 13.874999999999998, 13.95, 14.024999999999999, 14.1, 14.174999999999999, 14.249999999999998, 14.325, 14.399999999999999, 14.474999999999998, 14.549999999999999, 14.624999999999998, 14.7, 14.774999999999999, 14.849999999999998, 14.924999999999999, 14.999999999999998, 15.075, 15.149999999999999, 15.224999999999998, 15.299999999999999, 15.374999999999998, 15.45, 15.524999999999999, 15.599999999999998, 15.674999999999999, 15.749999999999998, 15.825, 15.899999999999999, 15.974999999999998, 16.05, 16.125, 16.2, 16.275, 16.349999999999998, 16.424999999999997, 16.5, 16.575, 16.65, 16.724999999999998, 16.799999999999997, 16.875, 16.95, 17.025, 17.099999999999998, 17.174999999999997, 17.25, 17.325, 17.4, 17.474999999999998, 17.549999999999997, 17.625, 17.7, 17.775, 17.849999999999998, 17.924999999999997, 18.0, 18.075, 18.15, 18.224999999999998, 18.299999999999997, 18.375, 18.45, 18.525, 18.599999999999998, 18.674999999999997, 18.75, 18.825, 18.9, 18.974999999999998, 19.049999999999997, 19.125, 19.2, 19.275, 19.349999999999998, 19.424999999999997, 19.5, 19.575, 19.65, 19.724999999999998, 19.799999999999997, 19.875, 19.95, 20.025, 20.099999999999998, 20.174999999999997, 20.25, 20.325, 20.4, 20.474999999999998, 20.549999999999997, 20.625, 20.7, 20.775, 20.849999999999998, 20.924999999999997, 21.0]}, ...(2 in all)]
  in  "dead time":dbl=3.7e-08
  out "Optical Depth":cluster{"Y":dbl[], "Y":dbl[]}[](graph) caption="XY Graph"
  out "RingBuffer offline far":dbl[][](array[numeric])
  out "RingBuffer aerosol far":dbl[][](array[numeric])
  in  "Weather":T3(tab)=enum."Pulse Energy (Micro Joule)"
  in  "Temperature (C)":dbl=15.0
  out "Temperature (C)":dbl(graph)=15.0
  in  "Pressure (mbar or hPa)":dbl=832.0
  out "Pressure (mb)":dbl(graph)=832.0
  out "Relative Humdity (%)":dbl(graph)=40.0
  out "Pulse Energy (Micro Joule)":T4(graph)={"Online Pulse Energy"=4.73832, "Pulse Energy Offline"=4.74074}
  out "?":cluster{"mean":dbl, "mean":dbl}(graph)={"mean"=nan, "mean"=nan}
  out "Index":i32=24
  out "Aerosol Smoothed":dbl[](array[numeric])=[729.1169811320754, 948.0320754716977, 1131.3245283018864, 1271.796226415094, 1331.5981132075472, 1313.6358490566035, 1265.418867924528, 1198.6924528301884, 1107.6830188679241, 1013.7018867924523, 927.6169811320751, 845.9471698113205, 778.2867924528299, 715.8622641509432, 646.4188679245282, 587.7962264150942, 533.5981132075472, 490.6924528301886, 456.9283018867924, 417.2113207547169, 386.4849056603773, 360.3716981132075, 330.45660377358496, 308.0886792452831, 283.9377358490567, 262.0886792452832, 250.83396226415107, 240.6547169811322, 222.27735849056614, 199.38113207547175, 186.7773584905661, 180.61698113207552, 163.4849056603774, 151.02264150943398, 151.63584905660377, 145.29622641509434, 133.6075471698113, 125.33396226415094, 118.55094339622642, 110.06981132075471, 100.8811320754717, 92.94716981132075, 88.70188679245283, 84.74905660377357, 81.54150943396225, 78.28679245283016, 73.92830188679241, 69.48490566037734, 66.83396226415093, 62.95660377358488, 57.654716981132054, 53.81509433962262, 49.50377358490564, 44.447169811320734, 38.34339622641509, 32.843396226415095, 32.62641509433962, 31.409433962264146, 28.73962264150943, 29.82452830188679, 30.29622641509434, 25.994339622641505, 24.71132075471698, 24.645283018867925, 35.116981132075466, 96.0132075471698, 260.5226415094339, 449.29622641509434, 510.8716981132075, 479.86226415094336, 447.60754716981126, 405.4, 300.45660377358496, 150.04150943396232, 45.09811320754716, 14.17358490566038, 12.881132075471701, 12.75849056603774, 9.805660377358492, 5.843396226415094, 3.9660377358490564, 6.569811320754717, 6.541509433962264, 4.362264150943396, 5.003773584905661, 6.29622641509434, 4.749056603773584, 4.333962264150943, 7.522641509433962, 6.2679245283018865, 3.3716981132075468, 3.6641509433962263, 2.6735849056603773, 5.8339622641509425, 8.192452830188678, 4.758490566037736, 3.843396226415094, 3.5886792452830187, 3.0698113207547166, 3.9660377358490564, 5.409433962264151, 6.1169811320754715, 3.749056603773585, 2.6075471698113204, 2.984905660377358, 1.7773584905660376, 2.9377358490566037, 4.1830188679245275, 5.20188679245283, 3.739622641509434, 2.6358490566037736, 5.135849056603773, 5.569811320754717, 3.7962264150943392, 5.475471698113208, 7.749056603773585, 8.277358490566037, 5.437735849056604, 4.088679245283019, 8.909433962264153, 27.239622641509428, 62.541509433962254, 71.92830188679244, 40.267924528301876, 10.937735849056603, 3.2867924528301886, 3.3999999999999995, 3.494339622641509, 8.777358490566039, 31.456603773584895, 68.67358490566036, 86.16415094339621, 71.19245283018866, 65.02264150943394, 139.9283018867925, 315.60754716981137, 428.80566037735844, 326.08867924528306, 132.99433962264155, 26.20188679245282, 3.022641509433962, 3.9094339622641505, 2.7962264150943392, 3.9, 5.824528301886792, 3.7867924528301886, 3.7207547169811317, 1.70188679245283, 0.21132075471698095, 1.7490566037735846, 1.7113207547169809, 0.6547169811320752, 2.2773584905660376, 0.09811320754716957, 1.7490566037735844, 7.3528301886792455, 3.9849056603773585, -0.628301886792453, -2.2698113207547173, -0.7132075471698116, 3.041509433962264, 4.286792452830189, 2.833962264150943, 0.8811320754716979, 2.4283018867924526, 4.418867924528302, 4.711320754716981, 4.192452830188679, 0.11698113207547145, 0.3999999999999999, 1.6641509433962263, 0.4283018867924527, 1.2584905660377357, -0.4867924528301888, 0.10754716981132062, 2.3999999999999995, 1.4188679245283016, 1.2679245283018865, 3.522641509433962, 1.6264150943396225, 0.022641509433962037, 2.0981132075471693, 4.843396226415094, 6.607547169811321, 4.456603773584906, 2.7301886792452827, 3.409433962264151, 3.8245283018867924, 0.8716981132075469, -0.17547169811320779, 1.1547169811320752, 1.5603773584905658, -0.20377358490566067, -0.08113207547169843, 1.6075471698113204, 1.541509433962264, 5.418867924528302, 4.60754716981132, 1.0603773584905658, 1.7962264150943392, 3.6075471698113204, 2.654716981132075, 1.984905660377358, 1.4094339622641505, 0.9943396226415091, 2.7679245283018865, 0.6452830188679244, 2.145283018867924, 3.50377358490566, 2.9188679245283016, 1.852830188679245, 1.2396226415094338, 1.5792452830188677, -0.36415094339622667, 0.1264150943396224, 2.343396226415094, 3.2679245283018865, 2.4471698113207543, 2.3150943396226413, 3.6830188679245284, 3.239622641509434, 5.909433962264152, 5.560377358490567, 1.9849056603773585, 1.3433962264150943, 1.6169811320754715, 2.2301886792452827, 0.9188679245283017, 0.10754716981132054, -0.43018867924528326, 2.324528301886792, 2.8999999999999995, 0.8433962264150942, 1.1169811320754715, 2.4, 2.4, 3.550943396226415, 4.607547169811321, 3.324528301886792, 3.343396226415094, 1.692452830188679, 0.7773584905660376, 3.1169811320754715, 3.324528301886792, 2.7018867924528296, 1.315094339622641, 0.6358490566037733, 1.5698113207547169, 1.0792452830188677, 1.852830188679245, 3.673584905660377, 4.8528301886792455, 3.9, 1.220754716981132, 1.3905660377358489, 3.2018867924528296, 2.6641509433962263, 2.126415094339622, 1.9566037735849053, 1.862264150943396, 4.409433962264151, 5.4, 2.20188679245283, -1.5811320754716984, -0.36415094339622667, 3.9377358490566037, 2.5509433962264145, -0.5245283018867927, -3.005660377358491, -2.109433962264151, 2.4754716981132074, 0.2584905660377357, -3.118867924528302, -1.2037735849056606, 2.494339622641509, 2.9471698113207543, 2.249056603773585]
  out "Off-Line  Bin Readings":dbl[](array[numeric])
  out "Off-Line Smoothed":dbl[](array[numeric])=[522.3783251231526, 656.013793103448, 764.5334975369453, 846.4940886699503, 880.2182266009847, 872.0999999999995, 844.1960591133, 803.0655172413788, 745.7133004926103, 683.2133004926105, 624.7231527093595, 572.1591133004925, 523.7231527093595, 478.5679802955664, 434.0778325123151, 394.5729064039408, 360.3832512315271, 331.01625615763544, 304.46699507389155, 279.356157635468, 258.7083743842365, 240.69605911330055, 221.18128078817745, 204.56551724137944, 190.41034482758633, 178.06551724137944, 168.4300492610838, 159.06551724137933, 148.343842364532, 136.17142857142858, 127.28226600985224, 121.45714285714287, 112.0162561576355, 104.17635467980298, 100.90049261083745, 95.77733990147783, 89.58522167487683, 83.62216748768473, 78.5704433497537, 73.28226600985221, 67.91527093596059, 63.1911330049261, 59.29211822660097, 56.64187192118224, 54.58275862068962, 50.94975369458125, 47.79458128078814, 46.33152709359602, 44.18128078817732, 41.907881773399005, 38.78965517241379, 35.7527093596059, 33.70837438423645, 30.501477832512307, 26.001477832512315, 22.245320197044336, 20.466995073891624, 19.762561576354678, 19.73054187192118, 19.087684729064037, 19.191133004926108, 18.15911330049261, 16.614778325123154, 16.402955665024635, 25.272413793103446, 71.3536945812808, 170.53103448275874, 259.0556650246307, 366.484236453202, 513.9078817733989, 543.4201970443349, 391.44236453201967, 216.82167487684728, 104.86108374384236, 31.035960591132987, 9.516256157635464, 8.205911330049256, 6.959605911330047, 5.427586206896551, 4.095073891625615, 3.0532019704433493, 3.2379310344827577, 2.8758620689655165, 2.6098522167487674, 3.1073891625615757, 2.5285714285714285, 1.7748768472906398, 2.097536945812807, 3.0408866995073884, 2.186206896551724, 1.5261083743842359, 2.3192118226600975, 2.0581280788177327, 1.920197044334975, 2.604926108374384, 2.0236453201970437, 1.4399014778325119, 0.5556650246305413, -0.11182266009852268, 0.5433497536945807, 1.6492610837438417, 2.2896551724137924, 2.1788177339901473, 1.4571428571428566, 0.8832512315270931, 1.1246305418719207, 1.523645320197044, 1.752709359605911, 2.782266009852216, 3.388177339901477, 2.718226600985221, 2.272413793103448, 2.299507389162561, 1.336453201970443, 1.784729064039408, 2.9029556650246295, 3.114778325123152, 2.272413793103447, 1.1467980295566498, 1.883251231527093, 7.8068965517241375, 18.708374384236457, 20.21330049261084, 10.73793103448276, 3.1640394088669943, 0.7305418719211818, 0.5975369458128074, 0.7625615763546794, 4.306896551724135, 16.257635467980293, 35.05320197044334, 48.83152709359604, 46.50886699507387, 41.33645320197043, 86.58768472906404, 188.32906403940893, 241.17635467980307, 173.07290640394098, 66.09753694581283, 11.96945812807882, 0.8931034482758615, 2.104926108374383, 1.804433497536945, 1.6344827586206894, 1.833990147783251, 1.154187192118226, 1.0162561576354674, 0.21330049261083692, -0.01330049261083794, 0.4719211822660093, 0.590147783251231, 0.29950738916256103, 0.3142857142857138, -0.2891625615763552, 0.8068965517241375, 2.235467980295566, 1.757635467980295, 0.6911330049261079, -1.1881773399014783, -0.973891625615764, 0.5729064039408862, 1.5113300492610833, 1.319211822660098, 1.27487684729064, 1.6197044334975366, 0.8487684729064036, 0.3561576354679798, 0.5039408866995069, 0.1270935960591128, 0.21330049261083694, 1.06551724137931, 0.2231527093596054, 0.22561576354679747, 0.21822660098522112, 0.8758620689655168, 1.944827586206896, 0.6714285714285709, 1.0556650246305412, 2.215763546798029, 1.2305418719211818, 0.3364532019704428, 0.37832512315270883, 1.4103448275862065, 2.4029556650246304, 2.1369458128078813, 1.5975369458128075, 1.4916256157635464, 1.1862068965517236, -0.2793103448275867, -0.19064039408867045, 0.5039408866995069, 0.46453201970443303, 0.07783251231527044, -0.2768472906403946, 0.48423645320196995, 1.3093596059113297, 1.5433497536945808, 0.5852216748768468, -0.5256157635467985, 0.5679802955665021, 1.5802955665024627, 0.4793103448275857, 0.6788177339901473, 1.3339901477832508, 0.17881773399014728, -0.4665024630541877, -0.17339901477832564, 1.2576354679802952, 1.6123152709359603, 0.5753694581280784, 0.25270935960591084, -0.20541871921182317, 0.2330049261083739, 0.5852216748768468, 0.5113300492610833, 0.5507389162561571, 0.0999999999999995, 0.25270935960591084, 1.0113300492610833, 0.9423645320197039, 0.1566502463054182, 1.0975369458128075, 1.425123152709359, 1.0950738916256153, 0.5999999999999995, -0.7497536945812813, -0.17832512315270987, 0.5088669950738911, -0.35812807881773445, -0.21773399014778372, 1.5039408866995068, 1.7600985221674872, 0.9694581280788173, 0.3980295566502458, 0.9571428571428567, 1.338916256157635, 1.713300492610837, 1.5310344827586204, 0.11724137931034433, 0.7699507389162557, 1.5261083743842359, 0.6344827586206891, 0.2231527093596054, -0.2620689655172419, 0.27980295566502417, 1.3068965517241375, 1.0310344827586202, 0.31182266009852166, 0.04088669950738866, 0.3463054187192113, 0.7231527093596053, 0.6394088669950734, 0.4817733990147778, -0.5182266009852221, -0.11674876847290683, 1.3512315270935957, 1.319211822660098, 1.1443349753694576, 0.19852216748768425, -0.2004926108374389, 0.651724137931034, 1.2748768472906398, 1.1467980295566496, -0.055172413793104, -0.31133004926108426, 0.5507389162561571, 0.17881773399014728, -0.028078817733990652, -1.2645320197044339, -0.9837438423645324, 1.1418719211822654, 0.003940886699506874, -1.5674876847290644, -1.079802955665025, 0.8709359605911327, 1.895566502463054, 1.1270935960591129]
  out "On-Line  Smoothed":dbl[](array[numeric])=[1181.6039408866995, 1595.7763546798028, 1887.4463054187188, 2081.1950738916253, 2211.852709359606, 2270.9167487684726, 2230.815763546798, 2091.8059113300487, 1892.4733990147777, 1680.4857142857136, 1483.475862068965, 1298.1088669950739, 1121.554679802956, 962.2886699507392, 830.1384236453205, 735.9980295566503, 667.9561576354681, 602.9044334975371, 539.8330049261085, 488.2221674876849, 442.0940886699509, 401.6975369458129, 366.26403940886706, 329.76896551724144, 300.07192118226595, 277.0399014778325, 250.36995073891615, 229.1088669950738, 209.86748768472904, 189.73940886699506, 178.67044334975367, 166.92660098522168, 149.23694581280787, 136.87487684729064, 128.70492610837437, 116.02758620689653, 107.57684729064039, 100.22463054187193, 89.764039408867, 81.18029556650248, 77.06206896551727, 71.84285714285716, 64.84532019704436, 56.798522167487704, 51.49064039408867, 52.12857142857143, 47.968472906403946, 43.4167487684729, 38.66305418719212, 33.07192118226601, 28.510344827586216, 30.53004926108375, 32.62364532019705, 27.148275862068974, 23.599014778325127, 18.012807881773405, 12.793596059113302, 12.276354679802957, 14.786206896551725, 14.483251231527095, 8.968472906403946, 7.783743842364538, 7.052216748768479, 3.692610837438429, 1.032512315270941, 0.9019704433497587, 4.766502463054193, 10.796059113300498, 19.926600985221675, 42.15812807881774, 69.4832512315271, 549.3822660098522, 2398.3674876847294, 4038.490640394089, 3415.8699507389156, 1777.5768472906404, 586.8724137931036, 101.78374384236454, 36.150738916256174, 7.264039408866999, -4.585714285714279, -2.2310344827586146, 1.116256157635473, -2.1768472906403886, -1.955172413793098, -2.275369458128073, -6.191625615763542, -5.361576354679798, -5.7433497536945755, -2.354187192118222, 0.8182266009852268, -0.4970443349753644, 1.1729064039408916, 2.071921182266015, -2.7704433497536876, -2.6448275862068895, 1.0571428571428623, -3.9453201970443303, -6.684236453201966, -4.7852216748768415, -7.634975369458122, -6.590640394088664, -6.822167487684723, -9.896059113300492, -6.201477832512314, -2.2630541871921133, -1.9551724137930984, -3.1300492610837383, -6.538916256157629, -4.750738916256152, 0.9167487684729115, -3.1472906403940826, -8.450246305418712, -5.753201970443344, -2.3541871921182214, -2.0783251231527045, -0.6891625615763496, 2.0694581280788227, 1.6926108374384286, -1.425615763546793, -0.26551724137930544, -0.6891625615763495, -6.642364532019698, -4.206403940886694, -1.5290640394088624, 0.20246305418719657, 0.5078817733990195, 1.3453201970443396, 9.712315270935964, 21.143349753694586, 34.87733990147784, 43.40935960591134, 45.09655172413794, 43.761576354679804, 43.81083743842365, 44.25418719211824, 30.73940886699508, 8.958620689655177, -5.223645320197039, -6.346798029556646, -1.5487684729063989, -4.011822660098517, -5.13251231527093, -1.0660098522167436, 0.48078817733990664, -3.2827586206896497, -5.433004926108369, -1.44532019704433, 2.074384236453207, -1.642364532019699, -2.9034482758620634, -1.7679802955664972, -2.0019704433497485, -1.662068965517236, -3.014285714285709, -0.38374384236452697, -1.302463054187187, -1.3615763546797979, 0.7689655172413845, 0.10394088669951254, -1.2802955665024578, 0.07931034482759136, 0.3699507389162613, -2.280295566502458, -2.9674876847290586, -3.7014778325123103, -5.3270935960591075, -3.6571428571428513, 0.24187192118227116, 2.086699507389168, 1.5990147783251285, -2.4600985221674825, -0.8738916256157585, 1.970935960591138, 1.4931034482758672, 0.8551724137931086, -0.04137931034482244, 0.9536945812807933, 0.5472906403940938, -1.9280788177339852, -2.903448275862064, -4.208866995073886, -1.418226600985216, 1.633497536945818, 1.5004926108374437, 2.150738916256163, 1.470935960591138, -0.36896551724137416, 0.6482758620689706, 0.4142857142857195, -1.1226600985221622, 0.655665024630547, -1.657142857142852, -2.9502463054187142, -3.1768472906403895, -2.6423645320196996, -3.206403940886694, -3.563546798029551, -1.1866995073891573, -3.218719211822654, -4.361576354679797, -3.9108374384236404, -2.536453201970438, 0.7886699507389213, 2.658128078817739, -0.1300492610837387, -1.0758620689655123, 1.1014778325123205, 2.8674876847290687, 3.4364532019704477, -0.10788177339900917, -3.2999999999999945, -3.428078817733985, -2.299999999999995, -0.5832512315270885, -1.2802955665024573, -1.2679802955664967, -1.4231527093596008, -2.053694581280783, 0.6926108374384288, 3.778817733990153, 3.9512315270936016, -2.147290640394083, -3.063546798029551, 1.2886699507389214, -0.2926108374384184, -3.0216748768472854, 1.1876847290640442, 2.4610837438423694, 1.1334975369458178, 0.6753694581280839, 1.025123152709365, 0.7911330049261136, -2.905911330049256, 0.3330049261083794, 2.158128078817739, -0.28768472906403425, -1.950246305418714, -0.8246305418719161, -0.7802955665024579, -1.3172413793103397, 2.091625615763552, -1.6201970443349696, -5.524137931034476, -1.2384236453201902, -0.2655172413793052, -0.7064039408866943, -1.2211822660098473, -1.5610837438423595, 0.6113300492610889, -1.1891625615763495, -1.1522167487684678, 2.340394088669956, 4.150738916256163, 3.1729064039408916, 0.9832512315270987, 0.7615763546798082, -2.780295566502457, -3.674384236453196, 0.9635467980295619, -1.0807881773398957, -0.5487684729063989, 1.2541871921182313, 1.884729064039414, 2.865024630541877, 0.8305418719211874, 3.99556650246306, 2.5620689655172475, -2.304926108374379, -0.9600985221674825, -0.7778325123152656, -1.5660098522167436, -0.15714285714285198, 0.884729064039414, -0.05123152709359097, -0.03891625615763039, 1.9167487684729114]
  out "On-Line Bin Readings":dbl[](array[numeric])=[1643.0, 2156.0, 2533.0, 2883.0, 3214.0, 3212.0, 3144.0, 2989.0, 2811.0, 2673.0, 2469.0, 2330.0, 1964.0, 1853.0, 1626.0, 1504.0, 1383.0, 1362.0, 1214.0, 1151.0, 1137.0, 1053.0, 1084.0, 1037.0, 958.0, 966.0, 886.0, 902.0, 892.0, 850.0, 774.0, 856.0, 793.0, 784.0, 792.0, 764.0, 725.0, 729.0, 661.0, 657.0, 722.0, 666.0, 643.0, 640.0, 709.0, 672.0, 644.0, 655.0, 702.0, 691.0, 697.0, 670.0, 625.0, 653.0, 649.0, 632.0, 644.0, 605.0, 684.0, 653.0, 599.0, 621.0, 595.0, 609.0, 615.0, 644.0, 649.0, 613.0, 611.0, 644.0, 612.0, 603.0, 624.0, 628.0, 648.0, 668.0, 685.0, 695.0, 719.0, 784.0, 747.0, 616.0, 625.0, 628.0, 620.0, 649.0, 629.0, 600.0, 597.0, 654.0, 671.0, 614.0, 641.0, 598.0, 594.0, 644.0, 612.0, 662.0, 608.0, 637.0, 629.0, 600.0, 631.0, 594.0, 652.0, 614.0, 645.0, 615.0, 630.0, 630.0, 577.0, 660.0, 596.0, 604.0, 585.0, 624.0, 614.0, 643.0, 619.0, 625.0, 585.0, 586.0, 615.0, 638.0, 598.0, 618.0, 636.0, 588.0, 644.0, 668.0, 698.0, 746.0, 858.0, 840.0, 809.0, 788.0, 820.0, 751.0, 681.0, 562.0, 641.0, 568.0, 633.0, 628.0, 621.0, 600.0, 620.0, 579.0, 623.0, 612.0, 604.0, 582.0, 664.0, 607.0, 607.0, 575.0, 609.0, 625.0, 634.0, 590.0, 611.0, 642.0, 605.0, 631.0, 623.0, 561.0, 598.0, 624.0, 630.0, 678.0, 642.0, 645.0, 578.0, 625.0, 586.0, 602.0, 621.0, 677.0, 574.0, 598.0, 624.0, 642.0, 604.0, 603.0, 620.0, 551.0, 594.0, 602.0, 602.0, 572.0, 594.0, 590.0, 643.0, 625.0, 602.0, 598.0, 624.0, 661.0, 641.0, 600.0, 605.0, 634.0, 624.0, 612.0, 652.0, 645.0, 545.0, 594.0, 643.0, 617.0, 609.0, 645.0, 579.0, 614.0, 642.0, 616.0, 619.0, 608.0, 595.0, 613.0, 664.0, 664.0, 626.0, 619.0, 701.0, 565.0, 620.0, 657.0, 647.0, 618.0, 615.0, 629.0, 604.0, 591.0, 623.0, 643.0, 602.0, 663.0, 612.0, 610.0, 634.0, 631.0, 571.0, 625.0, 590.0, 625.0, 621.0, 548.0, 614.0, 577.0, 665.0, 621.0, 589.0, 605.0, 623.0, 587.0, 614.0, 652.0, 602.0, 653.0, 595.0, 637.0, 627.0, 616.0, 619.0, 602.0, 574.0, 631.0, 688.0, 646.0, 585.0, 621.0, 614.0, 642.0, 606.0, 607.0, 611.0, 590.0, 572.0]
  out "Range Corrected Altitude Array":dbl[](array[numeric])=[5625.0, 22500.0, 50625.0, 90000.0, 140625.0, 202500.0, 275625.0, 360000.0, 455625.0, 562500.0, 680625.0, 810000.0, 950625.0, 1102500.0, 1265625.0, 1440000.0, 1625625.0, 1822500.0, 2030625.0, 2250000.0, 2480625.0, 2722500.0, 2975625.0, 3240000.0, 3515625.0, 3802500.0, 4100625.0, 4410000.0, 4730625.0, 5062500.0, 5405625.0, 5760000.0, 6125625.0, 6502500.0, 6890625.0, 7290000.0, 7700625.0, 8122500.0, 8555625.0, 9000000.0, 9455625.0, 9922500.0, 10400625.0, 10890000.0, 11390625.0, 11902500.0, 12425625.0, 12960000.0, 13505625.0, 14062500.0, 14630625.0, 15210000.0, 15800625.0, 16402500.0, 17015625.0, 17640000.0, 18275625.0, 18922500.0, 19580625.0, 20250000.0, 20930625.0, 21622500.0, 22325625.0, 23040000.0, 23765625.0, 24502500.0, 25250625.0, 26010000.0, 26780625.0, 27562500.0, 28355625.0, 29160000.0, 29975625.0, 30802500.0, 31640625.0, 32490000.0, 33350625.0, 34222500.0, 35105625.0, 36000000.0, 36905625.0, 37822500.0, 38750625.0, 39690000.0, 40640625.0, 41602500.0, 42575625.0, 43560000.0, 44555625.0, 45562500.0, 46580625.0, 47610000.0, 48650625.0, 49702500.0, 50765625.0, 51840000.0, 52925625.0, 54022500.0, 55130625.0, 56250000.0, 57380625.0, 58522500.0, 59675625.0, 60840000.0, 62015625.0, 63202500.0, 64400625.0, 65610000.0, 66830625.0, 68062500.0, 69305625.0, 70560000.0, 71825625.0, 73102500.0, 74390625.0, 75690000.0, 77000625.0, 78322500.0, 79655625.0, 81000000.0, 82355625.0, 83722500.0, 85100625.0, 86490000.0, 87890625.0, 89302500.0, 90725625.0, 92160000.0, 93605625.0, 95062500.0, 96530625.0, 98010000.0, 99500625.0, 101002500.0, 102515625.0, 104040000.0, 105575625.0, 107122500.0, 108680625.0, 110250000.0, 111830625.0, 113422500.0, 115025625.0, 116640000.0, 118265625.0, 119902500.0, 121550625.0, 123210000.0, 124880625.0, 126562500.0, 128255625.0, 129960000.0, 131675625.0, 133402500.0, 135140625.0, 136890000.0, 138650625.0, 140422500.0, 142205625.0, 144000000.0, 145805625.0, 147622500.0, 149450625.0, 151290000.0, 153140625.0, 155002500.0, 156875625.0, 158760000.0, 160655625.0, 162562500.0, 164480625.0, 166410000.0, 168350625.0, 170302500.0, 172265625.0, 174240000.0, 176225625.0, 178222500.0, 180230625.0, 182250000.0, 184280625.0, 186322500.0, 188375625.0, 190440000.0, 192515625.0, 194602500.0, 196700625.0, 198810000.0, 200930625.0, 203062500.0, 205205625.0, 207360000.0, 209525625.0, 211702500.0, 213890625.0, 216090000.0, 218300625.0, 220522500.0, 222755625.0, 225000000.0, 227255625.0, 229522500.0, 231800625.0, 234090000.0, 236390625.0, 238702500.0, 241025625.0, 243360000.0, 245705625.0, 248062500.0, 250430625.0, 252810000.0, 255200625.0, 257602500.0, 260015625.0, 262440000.0, 264875625.0, 267322500.0, 269780625.0, 272250000.0, 274730625.0, 277222500.0, 279725625.0, 282240000.0, 284765625.0, 287302500.0, 289850625.0, 292410000.0, 294980625.0, 297562500.0, 300155625.0, 302760000.0, 305375625.0, 308002500.0, 310640625.0, 313290000.0, 315950625.0, 318622500.0, 321305625.0, 324000000.0, 326705625.0, 329422500.0, 332150625.0, 334890000.0, 337640625.0, 340402500.0, 343175625.0, 345960000.0, 348755625.0, 351562500.0, 354380625.0, 357210000.0, 360050625.0, 362902500.0, 365765625.0, 368640000.0, 371525625.0, 374422500.0, 377330625.0, 380250000.0, 383180625.0, 386122500.0, 389075625.0, 392040000.0, 395015625.0, 398002500.0, 401000625.0, 404010000.0, 407030625.0, 410062500.0, 413105625.0, 416160000.0, 419225625.0, 422302500.0, 425390625.0, 428490000.0, 431600625.0, 434722500.0, 437855625.0, 441000000.0]
  out "Altitude Array (km)":dbl[](array[numeric])=[0.075, 0.15, 0.22499999999999998, 0.3, 0.375, 0.45, 0.5249999999999999, 0.6, 0.6749999999999999, 0.7499999999999999, 0.825, 0.8999999999999999, 0.9749999999999999, 1.05, 1.125, 1.2, 1.275, 1.3499999999999999, 1.4249999999999998, 1.5, 1.575, 1.65, 1.7249999999999999, 1.7999999999999998, 1.8749999999999998, 1.95, 2.025, 2.1, 2.1750000000000003, 2.25, 2.325, 2.4, 2.475, 2.5500000000000003, 2.625, 2.7, 2.775, 2.85, 2.9250000000000003, 3.0, 3.075, 3.15, 3.225, 3.3000000000000003, 3.375, 3.45, 3.525, 3.6, 3.675, 3.75, 3.825, 3.9, 3.975, 4.05, 4.125, 4.2, 4.275, 4.35, 4.425, 4.5, 4.575, 4.65, 4.725, 4.8, 4.875, 4.95, 5.025, 5.1, 5.175, 5.25, 5.325, 5.4, 5.475, 5.55, 5.625, 5.7, 5.775, 5.85, 5.925, 6.0, 6.075, 6.15, 6.225, 6.3, 6.375, 6.45, 6.525, 6.6, 6.675, 6.75, 6.825, 6.9, 6.975, 7.05, 7.125, 7.2, 7.2749999999999995, 7.35, 7.425, 7.5, 7.575, 7.6499999999999995, 7.725, 7.8, 7.875, 7.95, 8.024999999999999, 8.1, 8.174999999999999, 8.249999999999998, 8.325, 8.399999999999999, 8.475, 8.549999999999999, 8.624999999999998, 8.7, 8.774999999999999, 8.85, 8.924999999999999, 8.999999999999998, 9.075, 9.149999999999999, 9.225, 9.299999999999999, 9.374999999999998, 9.45, 9.524999999999999, 9.6, 9.674999999999999, 9.749999999999998, 9.825, 9.899999999999999, 9.975, 10.049999999999999, 10.124999999999998, 10.2, 10.274999999999999, 10.35, 10.424999999999999, 10.499999999999998, 10.575, 10.649999999999999, 10.725, 10.799999999999999, 10.874999999999998, 10.95, 11.024999999999999, 11.1, 11.174999999999999, 11.249999999999998, 11.325, 11.399999999999999, 11.475, 11.549999999999999, 11.624999999999998, 11.7, 11.774999999999999, 11.85, 11.924999999999999, 11.999999999999998, 12.075, 12.149999999999999, 12.225, 12.299999999999999, 12.374999999999998, 12.45, 12.524999999999999, 12.6, 12.674999999999999, 12.749999999999998, 12.825, 12.899999999999999, 12.975, 13.049999999999999, 13.124999999999998, 13.2, 13.274999999999999, 13.35, 13.424999999999999, 13.499999999999998, 13.575, 13.649999999999999, 13.725, 13.799999999999999, 13.874999999999998, 13.95, 14.024999999999999, 14.1, 14.174999999999999, 14.249999999999998, 14.325, 14.399999999999999, 14.474999999999998, 14.549999999999999, 14.624999999999998, 14.7, 14.774999999999999, 14.849999999999998, 14.924999999999999, 14.999999999999998, 15.075, 15.149999999999999, 15.224999999999998, 15.299999999999999, 15.374999999999998, 15.45, 15.524999999999999, 15.599999999999998, 15.674999999999999, 15.749999999999998, 15.825, 15.899999999999999, 15.974999999999998, 16.05, 16.125, 16.2, 16.275, 16.349999999999998, 16.424999999999997, 16.5, 16.575, 16.65, 16.724999999999998, 16.799999999999997, 16.875, 16.95, 17.025, 17.099999999999998, 17.174999999999997, 17.25, 17.325, 17.4, 17.474999999999998, 17.549999999999997, 17.625, 17.7, 17.775, 17.849999999999998, 17.924999999999997, 18.0, 18.075, 18.15, 18.224999999999998, 18.299999999999997, 18.375, 18.45, 18.525, 18.599999999999998, 18.674999999999997, 18.75, 18.825, 18.9, 18.974999999999998, 19.049999999999997, 19.125, 19.2, 19.275, 19.349999999999998, 19.424999999999997, 19.5, 19.575, 19.65, 19.724999999999998, 19.799999999999997, 19.875, 19.95, 20.025, 20.099999999999998, 20.174999999999997, 20.25, 20.325, 20.4, 20.474999999999998, 20.549999999999997, 20.625, 20.7, 20.775, 20.849999999999998, 20.924999999999997, 21.0]
  out "Offline Pulse Energy":dbl=4.7377714285714285
  out "Online Pulse Energy":dbl=4.73832
  in  "Instrument Control":T5(tab)=enum."DAQ"
  in  "ILX Address On":dbl=1.0 min=0.0 step=1.0
  in  "ILX Address Off":dbl=2.0 min=0.0 step=1.0
  in  "OnLineLD":dbl=169.7
  in  "OffLineLD":dbl=172.62
  in  "Pulse B Polarity":enum32{"Low", "High"}(ring)=enum."High"
  in  "Pulse A Delay(ns)":u32=1040 min=80 max=327600
  in  "Pulse B Delay(ns)":u32=170000 min=80 max=327600 step=1
  in  "Accumulation Delay(ns)":u32=10 min=10 max=1270 step=1
  in  "Sync Pulse Polarity":enum32{"Low", "High"}(ring)=enum."High"
  in  "Pulse A Polarity":enum32{"Low", "High"}(ring)=enum."High"
  in  "Number of Bins":u32=280 min=2 max=4095 step=1
  in  "Number of Accumulates":u32=10000 min=1 max=32767 step=1
  in  "Time Resolution Per Bin(ns)":u32=500 min=5 max=1063 step=1
  in  "Lambda On Set (nm)":dbl=828.198 format="%.5f"
  out "Lambda On Read (nm)":dbl=828.1979490082582 format="%.5f"
  out "Lambda Off Read (nm)":dbl=828.2973499058594 format="%.5f"
  in  "Lambda Off Set (nm)":dbl=828.29765 format="%#.5f"
  in  "Bristol In":i32=5
  out "Bristol Out":i32
  out "AB_DIF":dbl=-5.099174177303212e-05 format="%#_15g"
  out "NONAB_DIF":dbl=-0.000300094140584406 format="%#_15g"
  out "Wavelength Lock Online":bool=TRUE
  out "Wavelength Lock Offline":bool=TRUE
  in  "calculate absorption cross sections":bool
  in  "Smoothing Range":dbl=150.0
  in  "Total DIAL Integration Time (Minutes)":i32=3
  in  "Data Reads (number of loops)":i32=1
  in  "Total Aerosol Integration Time (Minutes)":dbl=0.5
  in  "Scalar Wait Time":u32
  out "Smoothed Bins":dbl=2.0
  in  "NewportIn":string
  in  "logging":bool
  out "Newport Device Key":string="1918-R 15120"
  in  "SampleSize":i32=2
  out "NewportRef":refnum<k24>
  in  "Switch Comm Port":refnum<visa-resource-name>="COM3"
  out "FF_On_Ref":refnum<file>
  out "FF_On_Ptr":i64=2832544 format="%.2p"
  out "FF_Off_Ref":refnum<file>
  out "FF_Off_Ptr":i64=1808056 format="%.2p"
  out "NF_On_Ref":refnum<file>
  out "NF_On_Ptr":i64=1808056 format="%.2p"
  out "NF_Off_Ref":refnum<file>
  out "NF_Off_Ptr":i64=1808056 format="%.2p"
  out "DataOpen":bool=TRUE
  out "File Path_Far Field (out)":string="C:\\Users\\H2ODial\\Desktop\\SharedTeleWVData\\160815FF\\17"
  out "File Path_Near Field (out)":string="C:\\Users\\H2ODial\\Desktop\\SharedTeleWVData\\160815NF\\17"
  in  "Data File DIR (in)":string="C:\\Users\\H2ODial\\Desktop\\SharedTeleWVData\\"
  in  "bins":u32=280 min=2 max=4095 step=1
  out "y offset":u32=10
  in  "ns scale":u32=500
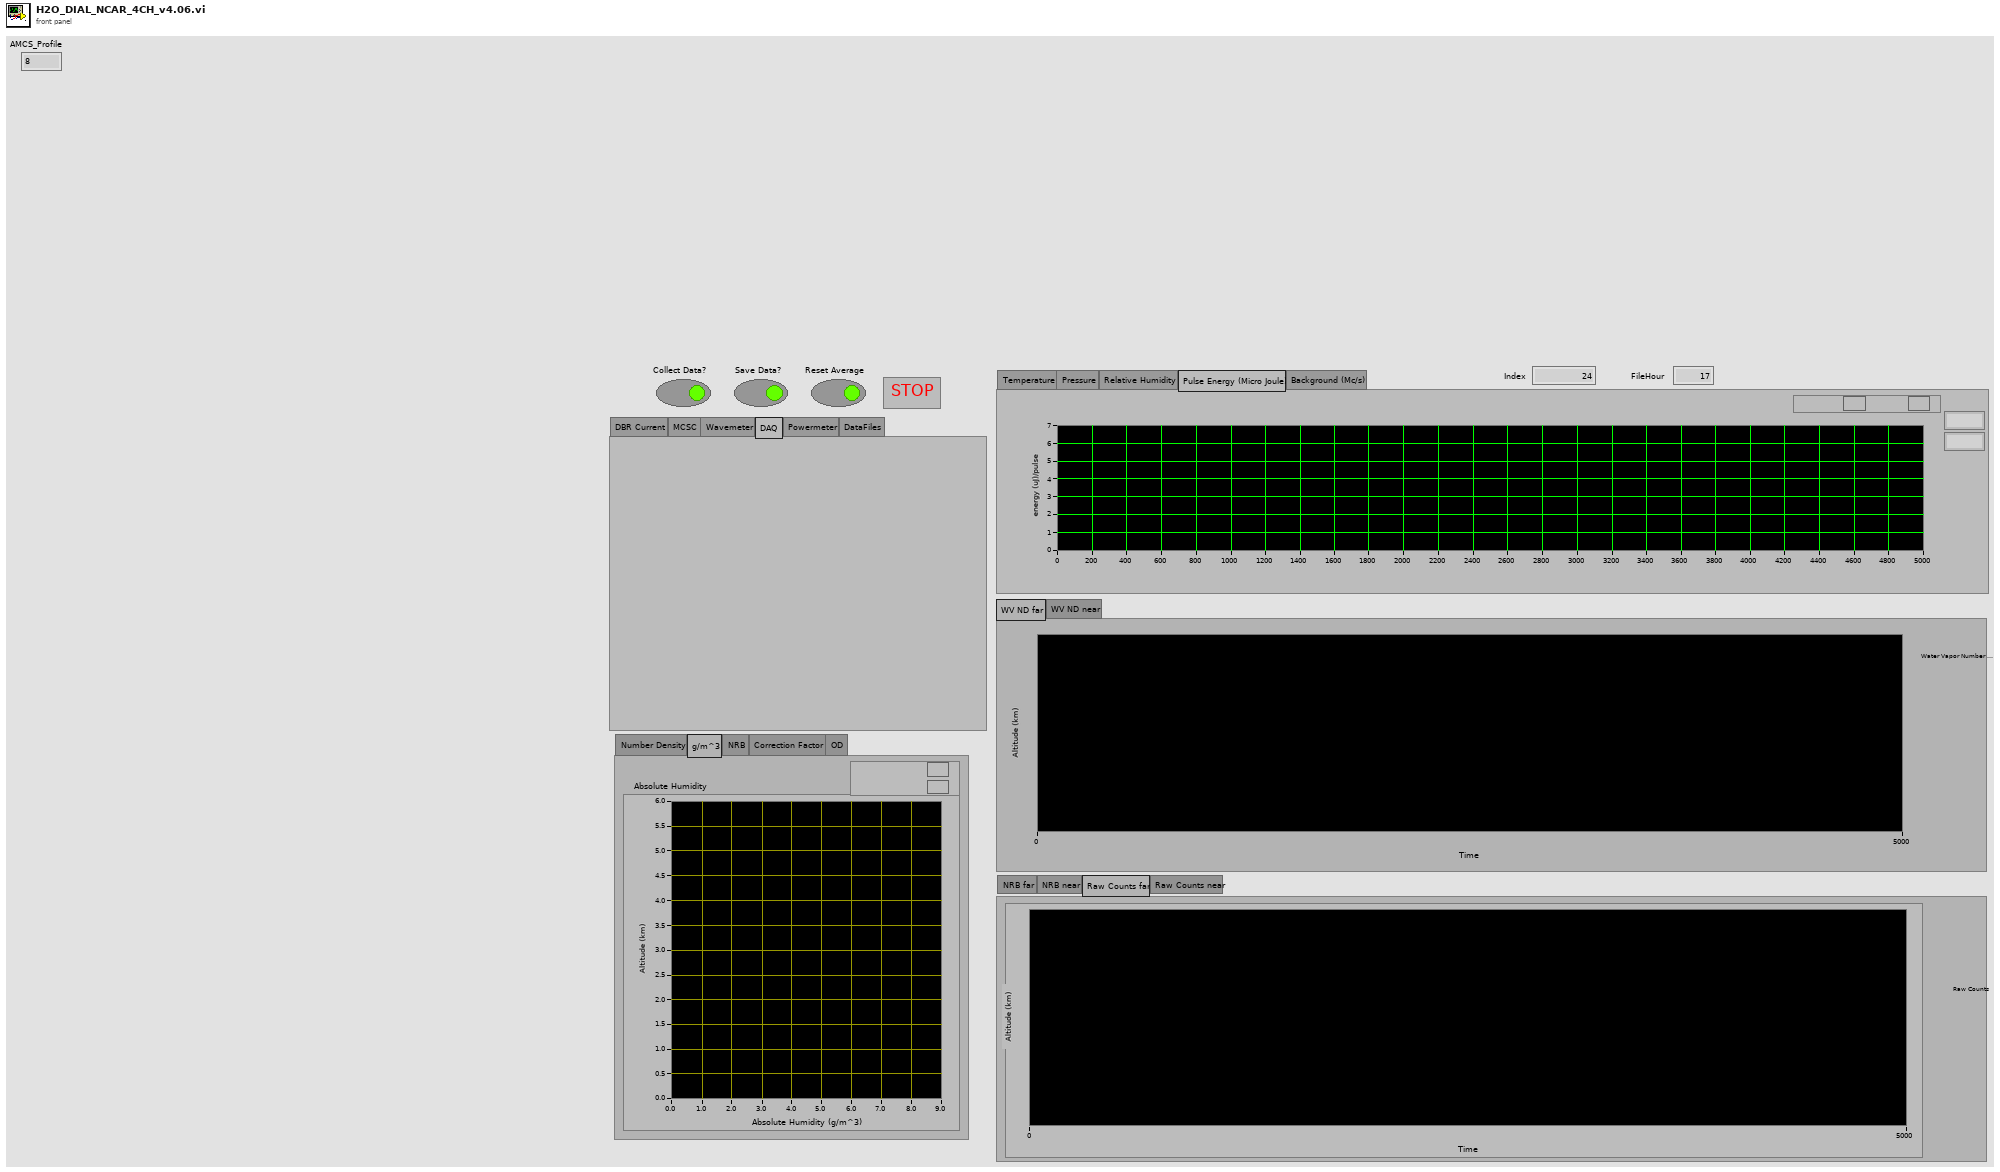
[diagram p1: front panel]
types:
  T1 = enum32{"NRB far", "NRB near", "Raw Counts far", "Raw Counts near"}
  T2 = enum32{"Number Density", "g/m^3", "NRB", "Correction Factor", "OD"}
  T3 = enum32{"Temperature", "Pressure", "Relative Humidity", "Pulse Energy (Micro Joule)", "Background (Mc/s)"}
  T4 = cluster{"Online Pulse Energy":dbl, "Pulse Energy Offline":dbl}
  T5 = enum32{"DBR Current", "MCSC", "Wavemeter", "DAQ", "Powermeter", "DataFiles"}
  T6 = enum16{"Initialize ILX", "Set ON T", "Set Off T", "Set ON I", "Set Off I", "Set On Lim", "Set Off Lim", "Read ILX", "TEC ON/OFF", "LASER ON/OFF", "Status?", "ILX OFF"}
  T7 = enum16{"open", "replace", "create", "open or create", "replace or create", "replace or create with confirmation"}
  T8 = typedef "LVDateTimeRec.ctl" = cluster{"fractional second":dbl, "second":i32, "minute":i32, "hour":i32, "day of month":i32, "month":i32, "year":i32, "day of week":i32, "day of year":i32, "DST":i32}
  T9 = cluster{"Online Pulse Energy":dbl, "Offline Pulse Energy":dbl}
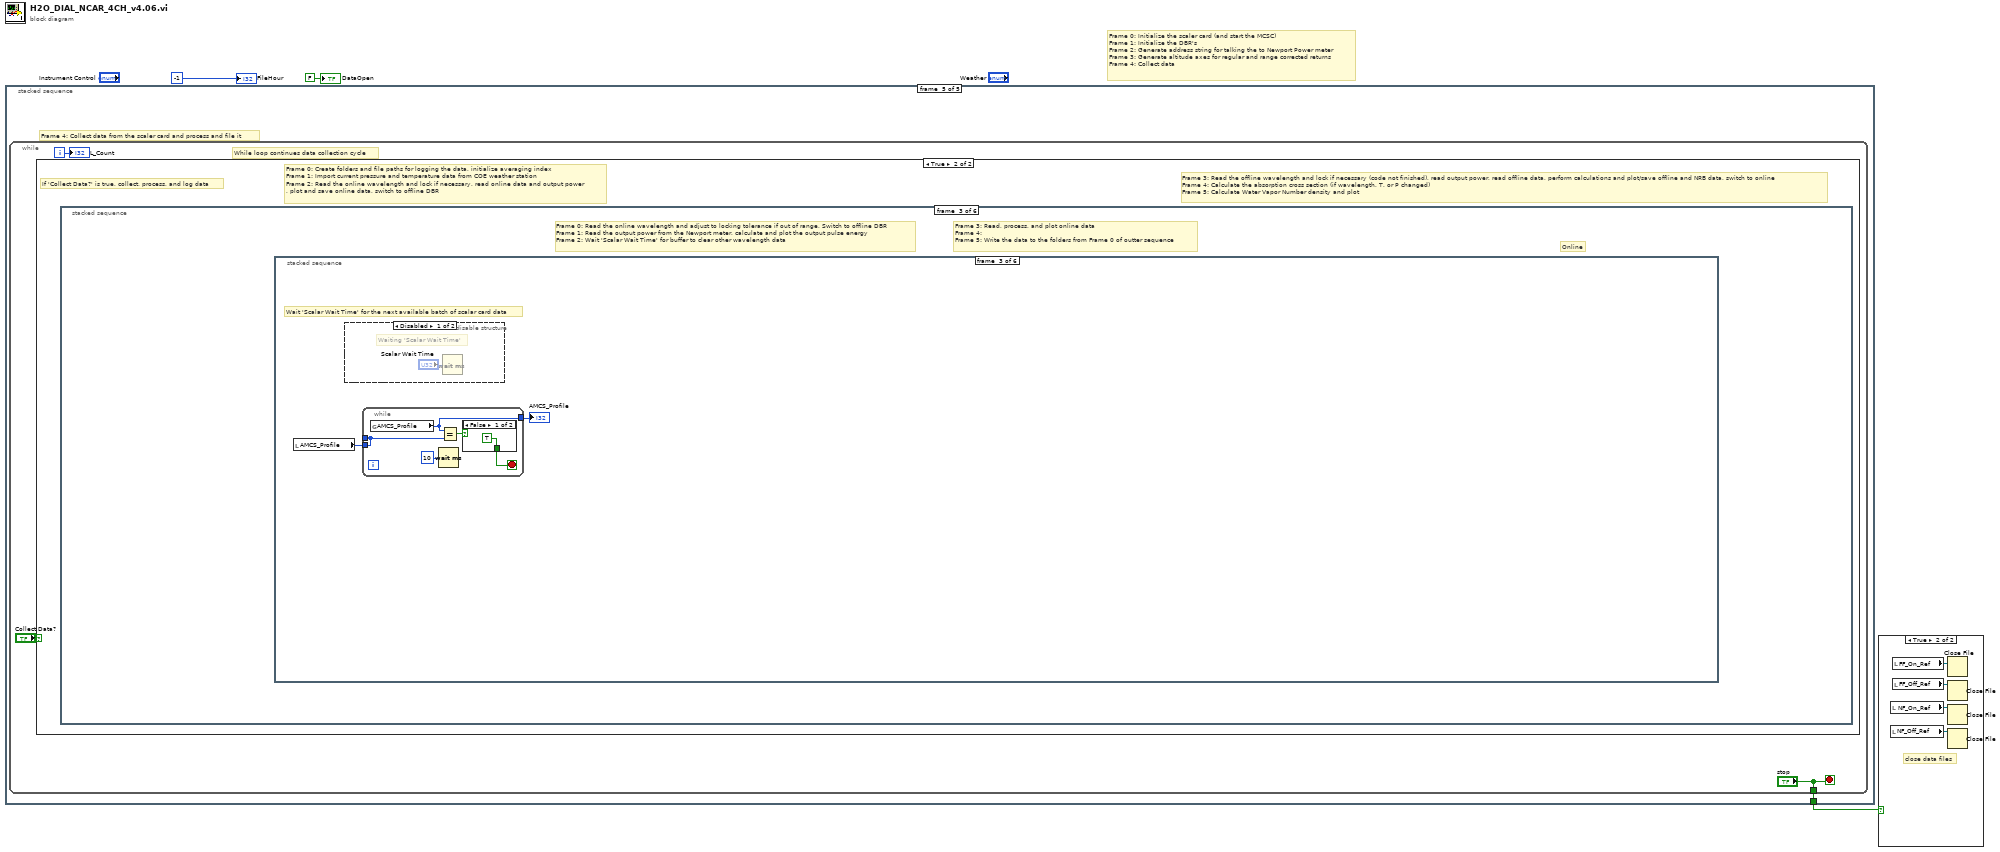
[diagram p0: block diagram]
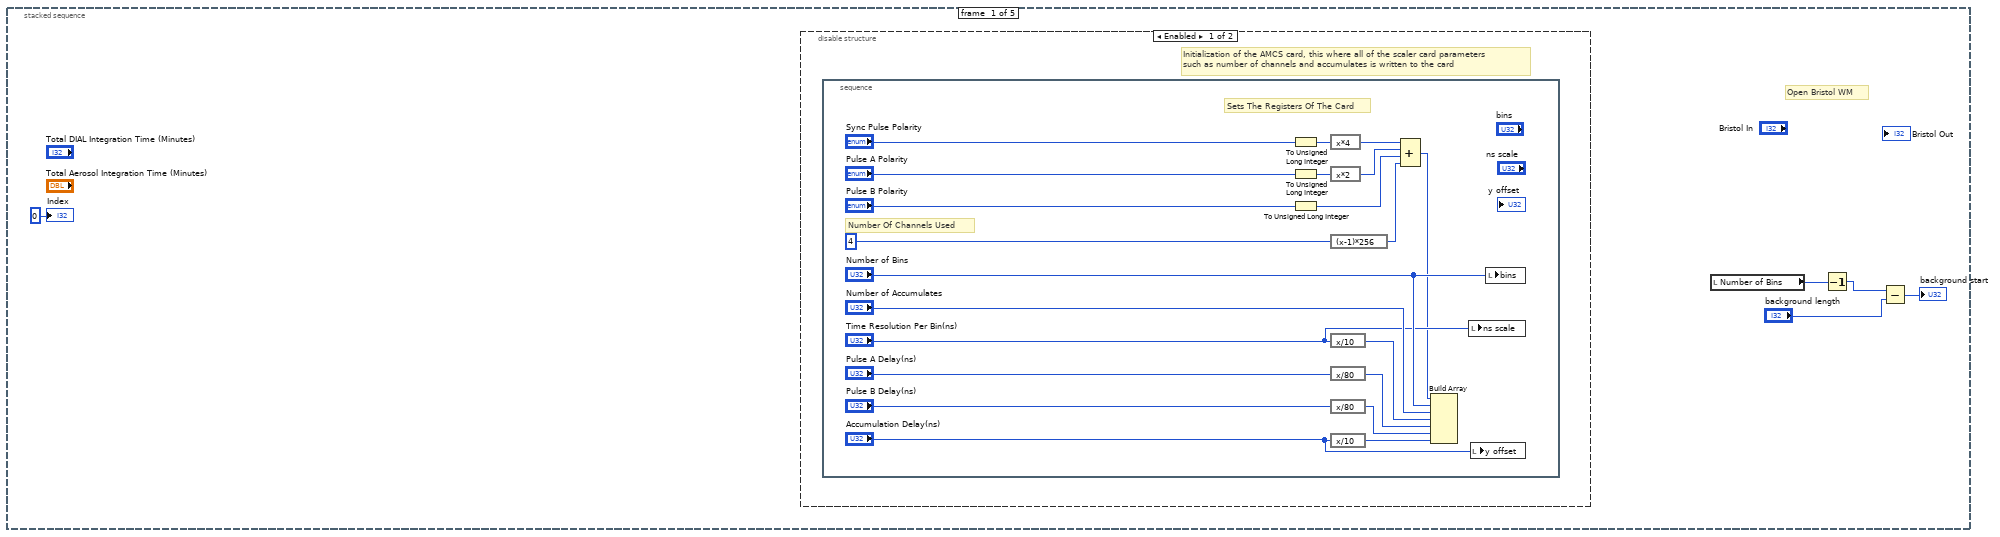
[diagram p3: hidden frame]
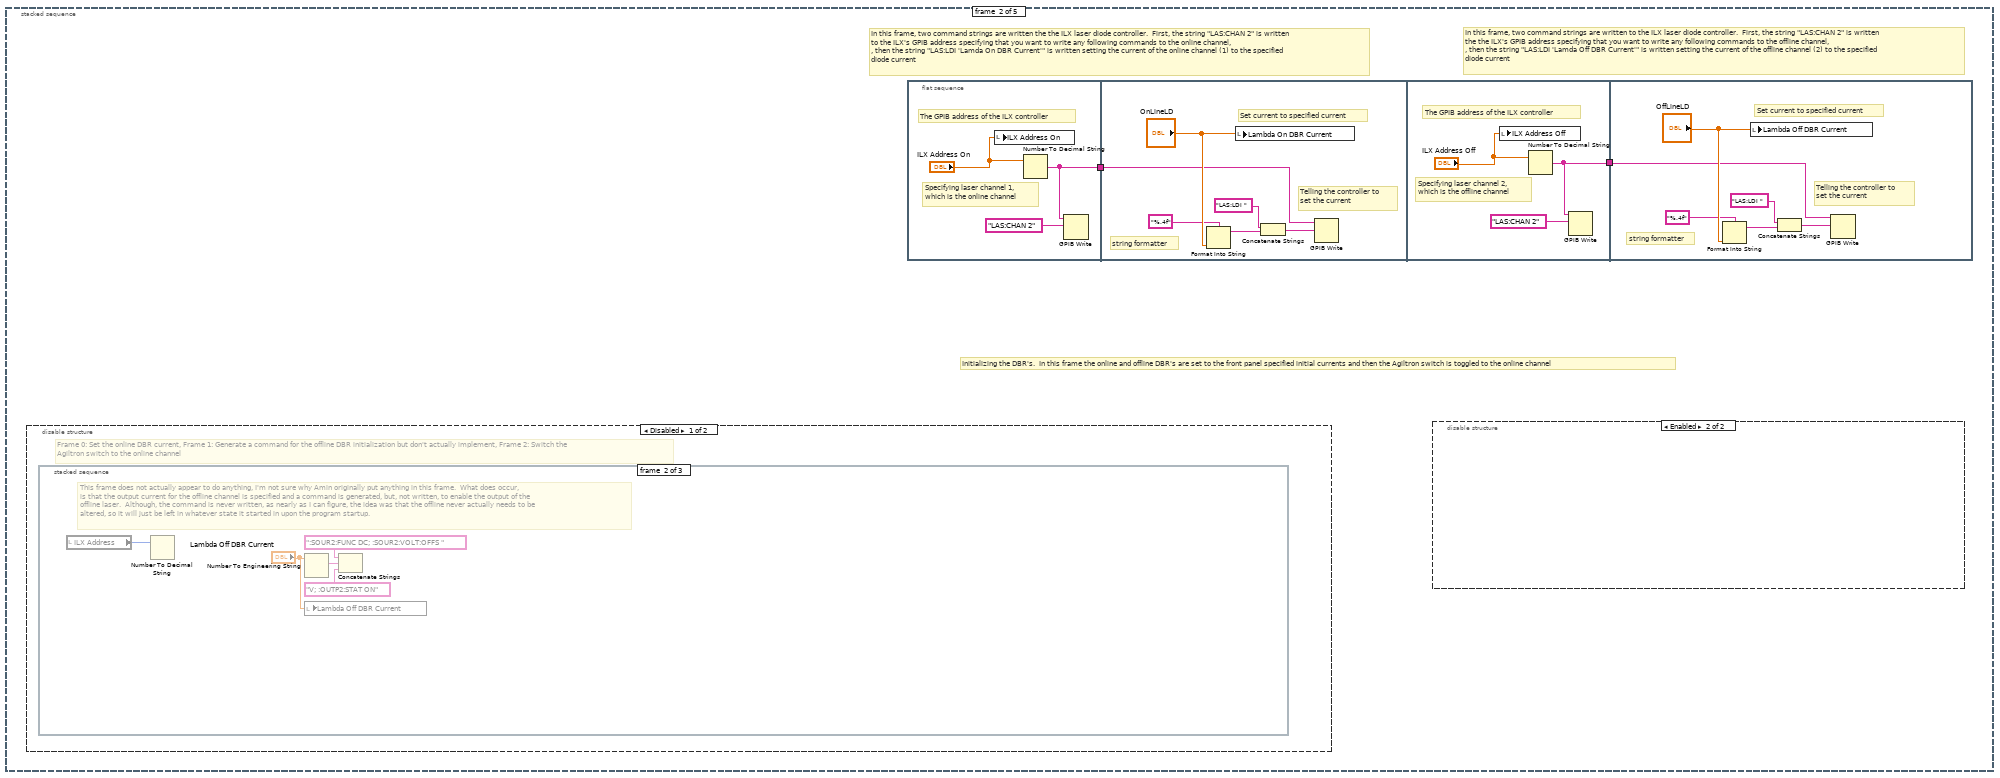
[diagram p5: hidden frame]
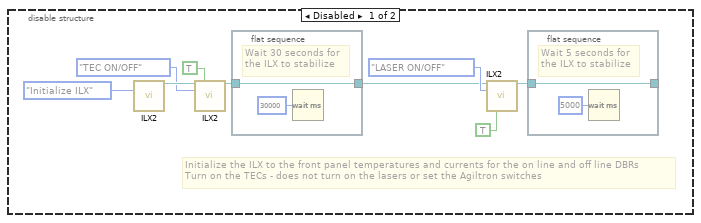
[diagram p6: hidden frame]
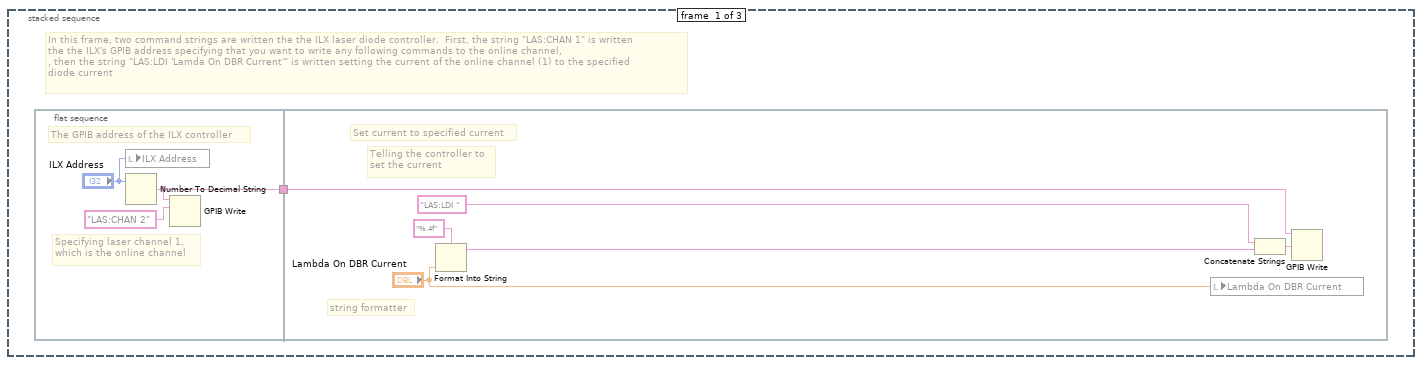
[diagram p7: hidden frame]
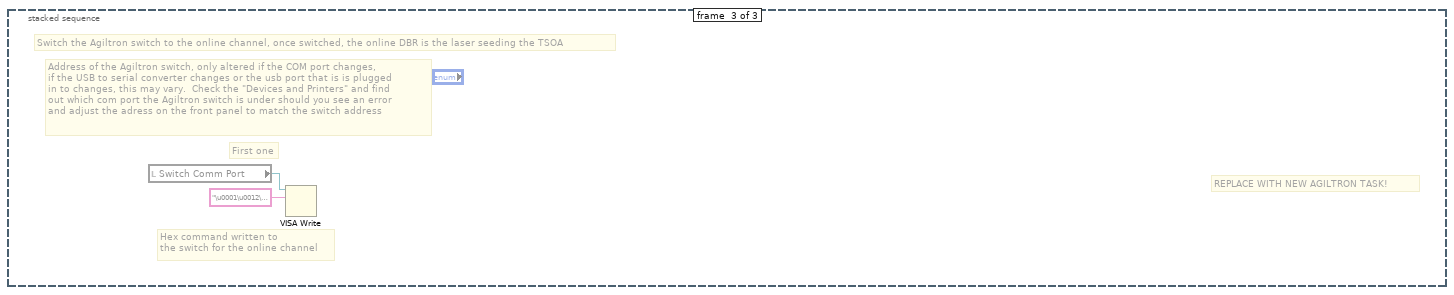
[diagram p8: hidden frame]
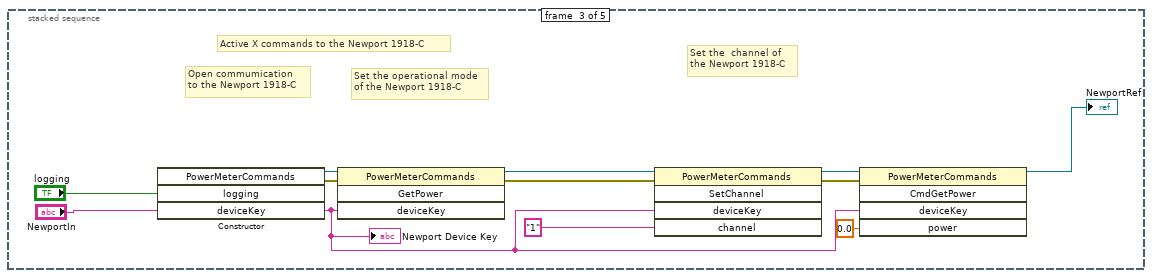
[diagram p10: hidden frame]
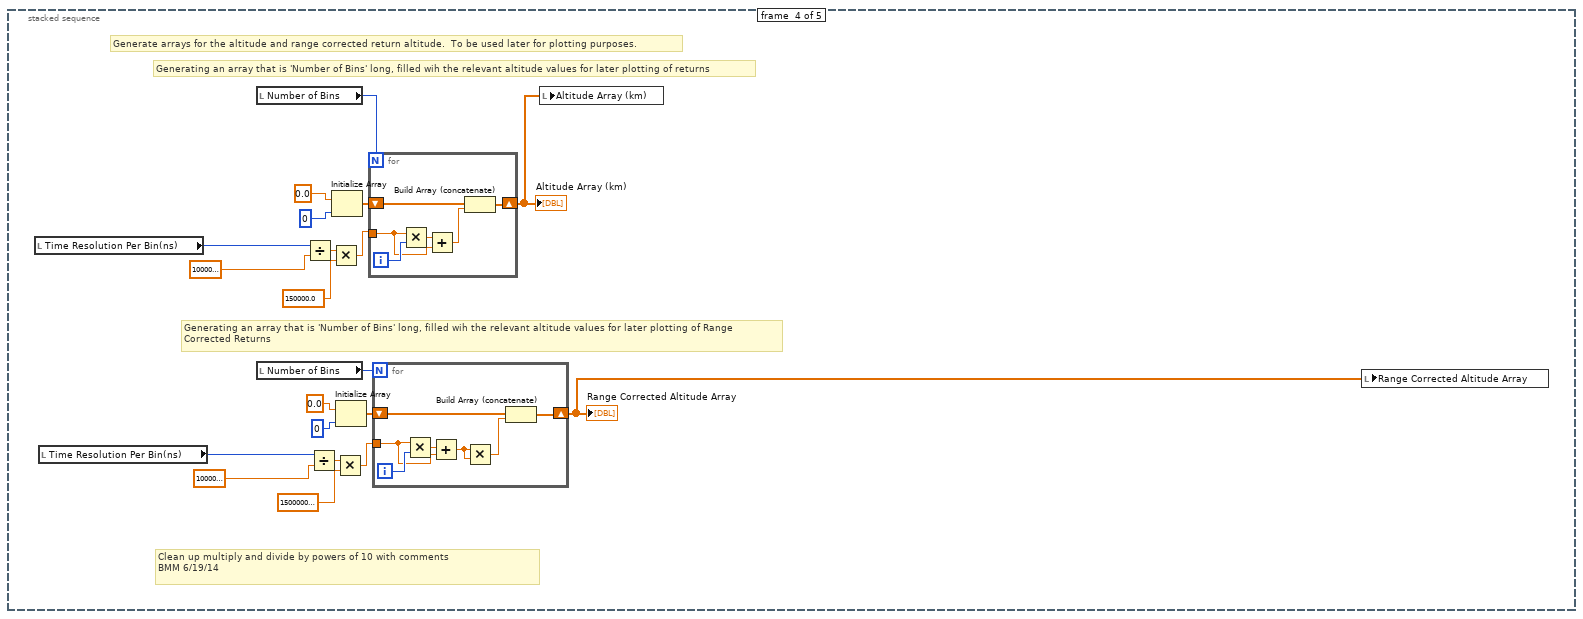
[diagram p11: hidden frame]
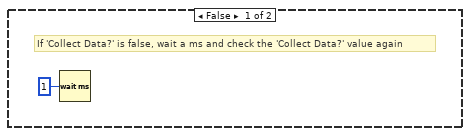
[diagram p12: hidden frame]
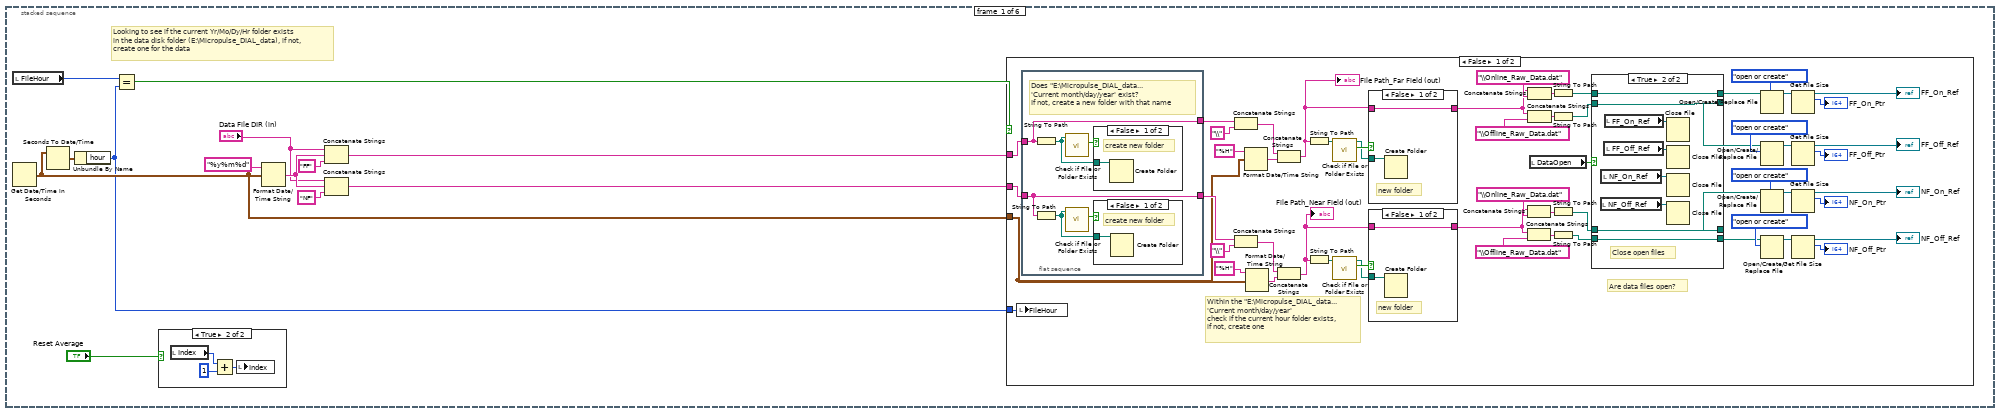
[diagram p13: hidden frame]
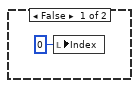
[diagram p20: hidden frame]
diagram:
  # "Frame 0: Initialize the scaler card (and start the MCSC)\nFrame 1: Initialize the DBR's\nFrame 2: Generate address string for talking the to Newport Power meter\nFrame 3: Generate altitude axes for regular and range corrected returns\nFrame 4: Collect data"
  n1 = stacked-sequence {
    tunnel: [_ _ _ _ w125] -> w3
    frame #0 {
      # "Open Bristol WM"
      n2 = disable-structure shown="Enabled" {
        frame Enabled {
          # "Initialization of the AMCS card, this where all of the scaler card parameters\nsuch as number of channels and accumulates is written to the card"
          n3 = stacked-sequence {
            frame #0 {
              # "Sets The Registers Of The Card"
              # "Number Of Channels Used"
              n4 = To Unsigned Long Integer(number="Sync Pulse Polarity") -> (unsigned 32bit integer=w9:u32)
              n5 = To Unsigned Long Integer(number="Pulse A Polarity") -> (unsigned 32bit integer=w13:u32)
              n6 = To Unsigned Long Integer(number="Pulse B Polarity") -> (unsigned 32bit integer=w11:u32)
              n7 = expression code="x*4"(w9) -> (w18:u32)
              n8 = expression code="x*2"(w13) -> (w17:u32)
              n9 = expression code="(x-1)*256"(u32 4 ("Number of Channels Used")) -> (w16:u32)
              n10 = expression code="x/10"("Time Resolution Per Bin(ns)") -> (w20:u32)
              n11 = expression code="x/80"("Pulse A Delay(ns)") -> (w27:u32)
              n12 = expression code="x/80"("Pulse B Delay(ns)") -> (w29:u32)
              n13 = expression code="x/10"("Accumulation Delay(ns)") -> (w28:u32)
              n14 = Compound Arithmetic op=ADD(w18, w17, w11, w16) -> (w15:u32)
              n15 = Build Array(w15, "Number of Bins", "Number of Accumulates", w20, w27, w29, w28) -> ()  [unwired: 1 out]
              n16 = local write "ns scale"("Time Resolution Per Bin(ns)") -> ()
              n17 = local write "y offset"("Accumulation Delay(ns)") -> ()
              n18 = local write "bins"("Number of Bins") -> ()
            }
          }
        }
        frame Disabled {
        }
      }
      n19 = local read "Number of Bins"() -> (w7:u32)
      n20 = Decrement(x=w7) -> (x-1=w6:u32)
      n21 = Subtract(x=w6, y="background length") -> (x-y=→"background start":u32)
      "Index" <- 0 ("Index")
    }
    frame #1 {
      # "In this frame, two command strings are written to the ILX laser diode controller.  First, the string \"LAS:CHAN 2\" is written\nthe the ILX's GPIB address specifying that you want to write any following commands to the offline channel,\n, then the string \"LAS:LDI 'Lamda Off DBR Current'\" is written setting the current of the offline channel (2) to the specified \ndiode current"
      # "In this frame, two command strings are written the the ILX laser diode controller.  First, the string \"LAS:CHAN 2\" is written\nto the ILX's GPIB address specifying that you want to write any following commands to the online channel,\n, then the string \"LAS:LDI 'Lamda On DBR Current'\" is written setting the current of the online channel (1) to the specified \ndiode current"
      # "Initializing the DBR's.  In this frame the online and offline DBR's are set to the front panel specified initial currents and then the Agiltron switch is toggled to the online channel"
      n22 = disable-structure shown="Disabled" {
        frame Disabled {
          # "Frame 0: Set the online DBR current, Frame 1: Generate a command for the offline DBR initialization but don't actually implement, Frame 2: Switch the \nAgiltron switch to the online channel"
          n23 = stacked-sequence {
            frame #0 {
              # "In this frame, two command strings are written the the ILX laser diode controller.  First, the string \"LAS:CHAN 1\" is written\nthe the ILX's GPIB address specifying that you want to write any following commands to the online channel,\n, then the string \"LAS:LDI 'Lamda On DBR Current'\" is written setting the current of the online channel (1) to the specified \ndiode current"
              n24 = flat-sequence {
                tunnel: [w65] -> w63
                tunnel: w63 -> [w67]
                frame #0 {
                  # "The GPIB address of the ILX controller"
                  # "Specifying laser channel 1,\nwhich is the online channel"
                  n25 = local write "ILX Address"("ILX Address") -> ()
                  n26 = Number To Decimal String(number="ILX Address") -> (decimal integer string=w65:string)  [unwired: 1 in]
                  n27 = GPIB Write(0:w65, 1:"LAS:CHAN 2") -> ()  [unwired: 3 in, 2 out]
                }
                frame #1 {
                  # "Telling the controller to\nset the current"
                  # "string formatter"
                  # "Set current to specified current"
                  n28 = Format Into String(format string="%.4f" ("Format String"), "Lambda On DBR Current") -> (resulting string=w70:string)  [unwired: 2 in, 1 out]
                  n29 = local write "Lambda On DBR Current"("Lambda On DBR Current") -> ()
                  n30 = Concatenate Strings("LAS:LDI ", w70) -> (w71:string)
                  n31 = GPIB Write(0:w67, 1:w71) -> ()  [unwired: 3 in, 2 out]
                }
              }
            }
            frame #1 {
              # "This frame does not actually appear to do anything, I'm not sure why Amin originally put anything in this frame.  What does occur, \nis that the output current for the offline channel is specified and a command is generated, but, not written, to enable the output of the\noffline laser.  Although, the command is never written, as nearly as I can figure, the idea was that the offline never actually needs to be \naltered, so it will just be left in whatever state it started in upon the program startup."
              n32 = local read "ILX Address"() -> (w73:i32)
              n33 = Number To Decimal String(number=w73) -> ()  [unwired: 1 in, 1 out]
              n34 = Number To Engineering String(4:"Lambda Off DBR Current") -> (0:w77:string)  [unwired: 3 in]
              n35 = local write "Lambda Off DBR Current"("Lambda Off DBR Current") -> ()
              n36 = Concatenate Strings(":SOUR2:FUNC DC; :SOUR2:VOLT:OFFS ", w77, "V; :OUTP2:STAT ON") -> ()  [unwired: 1 out]
            }
            frame #2 {
              # "REPLACE WITH NEW AGILTRON TASK!"
              # "First one"
              # "Address of the Agiltron switch, only altered if the COM port changes,\nif the USB to serial converter changes or the usb port that is is plugged\nin to changes, this may vary.  Check the \"Devices and Printers\" and find \nout which com port the Agiltron switch is under should you see an error \nand adjust the adress on the front panel to match the switch address"
              # "Hex command written to \nthe switch for the online channel"
              # "Switch the Agiltron switch to the online channel, once switched, the online DBR is the laser seeding the TSOA"
              n37 = local read "Switch Comm Port"() -> (w78:refnum<visa-resource-name>)
              n38 = VISA Write(VISA resource name=w78, write buffer="\u0001\u0012\u0000\u0002") -> ()  [unwired: 1 in, 3 out]
            }
          }
        }
        frame Enabled {
        }
      }
      n39 = flat-sequence {
        tunnel: [w33] -> w31
        tunnel: w31 -> [w35]
        tunnel: [w41] -> w30
        tunnel: w30 -> [w44]
        frame #0 {
          # "The GPIB address of the ILX controller"
          # "Specifying laser channel 1,\nwhich is the online channel"
          n40 = local write "ILX Address On"("ILX Address On") -> ()
          n41 = Number To Decimal String(number="ILX Address On") -> (decimal integer string=w33:string)  [unwired: 1 in]
          n42 = GPIB Write(0:w33, 1:"LAS:CHAN 2") -> ()  [unwired: 3 in, 2 out]
        }
        frame #1 {
          # "Telling the controller to\nset the current"
          # "string formatter"
          # "Set current to specified current"
          n43 = Format Into String(format string="%.4f" ("Format String"), "OnLineLD") -> (resulting string=w38:string)  [unwired: 2 in, 1 out]
          n44 = local write "Lambda On DBR Current"("OnLineLD") -> ()
          n45 = Concatenate Strings("LAS:LDI ", w38) -> (w39:string)
          n46 = GPIB Write(0:w35, 1:w39) -> ()  [unwired: 3 in, 2 out]
        }
        frame #2 {
          # "The GPIB address of the ILX controller"
          # "Specifying laser channel 2,\nwhich is the offline channel"
          n47 = local write "ILX Address Off"("ILX Address Off") -> ()
          n48 = Number To Decimal String(number="ILX Address Off") -> (decimal integer string=w41:string)  [unwired: 1 in]
          n49 = GPIB Write(0:w41, 1:"LAS:CHAN 2") -> ()  [unwired: 3 in, 2 out]
        }
        frame #3 {
          # "Telling the controller to\nset the current"
          # "string formatter"
          # "Set current to specified current"
          n50 = Format Into String(format string="%.4f" ("Format String"), "OffLineLD") -> (resulting string=w47:string)  [unwired: 2 in, 1 out]
          n51 = local write "Lambda Off DBR Current"("OffLineLD") -> ()
          n52 = Concatenate Strings("LAS:LDI ", w47) -> (w48:string)
          n53 = GPIB Write(0:w44, 1:w48) -> ()  [unwired: 3 in, 2 out]
        }
      }
      n54 = disable-structure shown="Enabled" {
        frame Disabled {
          # "Initialize the ILX to the front panel temperatures and currents for the on line and off line DBRs\nTurn on the TECs - does not turn on the lasers or set the Agiltron switches"
          n55 = call "ILX2.vi"("ILX Command"=T6."Initialize ILX") -> ("Device Out"=w57:refnum<visa-resource-name>)  [unwired: 10 in, 4 out]
          n56 = call "ILX2.vi"("Device In"=w57, "TEC Control"=TRUE, "ILX Command"=T6."TEC ON/OFF") -> ("Device Out"=w54:refnum<visa-resource-name>)  [unwired: 8 in, 4 out]
          n57 = flat-sequence {
            tunnel: w54 -> [w61]
            tunnel: [w61] -> w51
            frame #0 {
              # "Wait 30 seconds for\nthe ILX to stabilize"
              n58 = Wait (ms)(milliseconds to wait=u32 30000) -> ()  [unwired: 1 out]
            }
          }
          n59 = call "ILX2.vi"("Device In"=w51, "ILX Command"=T6."LASER ON/OFF", "Laser Control"=TRUE ("TEC Control")) -> ("Device Out"=w50:refnum<visa-resource-name>)  [unwired: 8 in, 4 out]
          n60 = flat-sequence {
            tunnel: w50 -> [w59]
            tunnel: [w59] -> _
            frame #0 {
              # "Wait 5 seconds for\nthe ILX to stabilize"
              n61 = Wait (ms)(milliseconds to wait=u32 5000) -> ()  [unwired: 1 out]
            }
          }
        }
        frame Enabled {
        }
      }
    }
    frame #2 {
      # "Active X commands to the Newport 1918-C"
      # "Set the  channel of\nthe Newport 1918-C"
      # "Set the operational mode\nof the Newport 1918-C"
      # "Open commumication\nto the Newport 1918-C"
      n62 = constructor class="PowerMeterCommands"("logging"="logging", "deviceKey"="NewportIn") -> (reference out=w91:refnum<k24>, error out=w88:errorcluster, "deviceKey"=w83:string)  [unwired: 3 in, 2 out]
      "Newport Device Key" <- w83
      n63 = invoke class="PowerMeterCommands" method="GetPower"(reference=w91, error in=w88, "deviceKey"=w83) -> (reference out=w90:refnum<k24>, error out=w87:errorcluster)  [unwired: 1 in, 2 out]
      n64 = invoke class="PowerMeterCommands" method="SetChannel"(reference=w90, error in=w87, "deviceKey"=w83, "channel"="1") -> (reference out=w84:refnum<k24>, error out=w86:errorcluster)  [unwired: 1 in, 3 out]
      n65 = invoke class="PowerMeterCommands" method="CmdGetPower"(reference=w84, error in=w86, "deviceKey"=w83, "power"=sgl 0.0) -> (reference out=→"NewportRef":refnum<k24>)  [unwired: 1 in, 4 out]
    }
    frame #3 {
      # "Clean up multiply and divide by powers of 10 with comments\nBMM 6/19/14"
      # "Generating an array that is 'Number of Bins' long, filled wih the relevant altitude values for later plotting of Range \nCorrected Returns"
      # "Generating an array that is 'Number of Bins' long, filled wih the relevant altitude values for later plotting of returns"
      # "Generate arrays for the altitude and range corrected return altitude.  To be used later for plotting purposes."
      n66 = local read "Time Resolution Per Bin(ns)"() -> (w104:u32)
      n67 = local read "Time Resolution Per Bin(ns)"() -> (w94:u32)
      n68 = local read "Number of Bins"() -> (w107:u32)
      n69 = local read "Number of Bins"() -> (w97:u32)
      n70 = Divide(x=w104, y=1000000000.0) -> (x/y=w102:dbl)
      n71 = Divide(x=w94, y=1000000000.0) -> (x/y=w92:dbl)
      n72 = Multiply(x=w102, y=150000.0) -> (x*y=w105:dbl)
      n73 = Initialize Array(0.0, 0) -> (w110:dbl[])
      n74 = Multiply(x=w92, y=150000000.0) -> (x*y=w95:dbl)
      n75 = Initialize Array(0.0, 0) -> (w100:dbl[])
      n76 = for {
        N: w107 -> [_]
        shift-right: [w123] -> w108
        shift-left: w110 -> [w124]
        tunnel: w105 -> [w120]
        i -> [w122]
        n77 = Multiply(x=w120, y=w122) -> (x*y=w121:dbl)
        n78 = Add(x=w121, y=w120) -> (x+y=w119:dbl)
        n79 = Build Array (concatenate)(w124, w119) -> (w123:dbl[])
      }
      "Altitude Array (km)" <- w108
      n80 = for {
        N: w97 -> [_]
        shift-right: [w117] -> w98
        shift-left: w100 -> [w118]
        tunnel: w95 -> [w113]
        i -> [w116]
        n81 = Multiply(x=w113, y=w116) -> (x*y=w114:dbl)
        n82 = Add(x=w114, y=w113) -> (x+y=w112:dbl)
        n83 = Multiply(x=w112, y=w112) -> (x*y=w115:dbl)
        n84 = Build Array (concatenate)(w118, w115) -> (w117:dbl[])
      }
      "Range Corrected Altitude Array" <- w98
      n85 = local write "Altitude Array (km)"(w108) -> ()
      n86 = local write "Range Corrected Altitude Array"(w98) -> ()
    }
    frame #4 {
      # "Frame 4: Collect data from the scaler card and process and file it"
      n87 = while {
        tunnel: ["stop"] -> w125
        i -> [w126]
        stop <- "stop" stop-if-true
        # "While loop continues data collection cycle"
        n88 = case shown="True" "Collect Data?" {
          frame False {
            # "If 'Collect Data?' is false, wait a ms and check the 'Collect Data?' value again"
            n89 = Wait (ms)(milliseconds to wait=u32 1) -> ()  [unwired: 1 out]
          }
          frame True {
            # "Frame 3: Read the offline wavelength and lock if necessary (code not finished), read output power, read offline data, perform calculations and plot/save offline and NRB data, switch to online\nFrame 4: Calculate the absorption cross section (if wavelength, T, or P changed)\nFrame 5: Calculate Water Vapor Number density and plot"
            # "Frame 0: Create folders and file paths for logging the data, initialize averaging index\nFrame 1: Import current pressure and temperature data from COE weather station\nFrame 2: Read the online wavelength and lock if necessary, read online data and output power\n, plot and save online data, switch to offline DBR"
            # "If 'Collect Data?' is true, collect, process, and log data"
            n90 = stacked-sequence {
              frame #0 {
                # "Looking to see if the current Yr/Mo/Dy/Hr folder exists\nin the data disk folder (E:\\Micropulse_DIAL_data), if not,\ncreate one for the data"
                n91 = local read "FileHour"() -> (w139:i32)
                n92 = Get Date/Time In Seconds() -> (seconds since 1Jan1904=w131:timestamp)
                n93 = Seconds To Date/Time(time stamp (now)=w131) -> (date time rec=w141:T8)  [unwired: 1 in]
                n94 = Unbundle By Name(w141) -> ("hour"=w130:i32)
                n95 = Equal?(x=w139, y=w130) -> (x = y?=w140:bool)
                n96 = case shown="True" "Reset Average" {
                  frame False {
                    n97 = local write "Index"(0 ("Index")) -> ()
                  }
                  frame True {
                    n98 = local read "Index"() -> (w229:i32)
                    n99 = Add(x=w229, y=1) -> (x+y=w228:i32)
                    n100 = local write "Index"(w228) -> ()
                  }
                }
                n101 = Format Date/Time String(time format string (%c)="%y%m%d", seconds (now)=w131) -> (date/time string=w135:string)  [unwired: 1 in]
                n102 = Concatenate Strings("Data File DIR (in)", w135, "FF" ("string")) -> (w137:string)
                n103 = Concatenate Strings("Data File DIR (in)", w135, "NF" ("string")) -> (w132:string)
                n104 = case shown="False" w140 {
                  tunnel: w137 -> [w199 _]
                  tunnel: w132 -> [w198 _]
                  tunnel: w131 -> [w185 _]
                  tunnel: w130 -> [w161 _]
                  frame False {
                    # "Are data files open?"
                    # "Within the \"E:\\Micropulse_DIAL_data...\n'Current month/day/year' \ncheck if the current hour folder exists,\nif not, create one"
                    n105 = local write "FileHour"(w161) -> ()
                    n106 = flat-sequence {
                      tunnel: [w219] -> w186
                      tunnel: w199 -> [w218]
                      tunnel: w198 -> [w219]
                      tunnel: [w218] -> w187
                      frame #0 {
                        # "Does \"E:\\Micropulse_DIAL_data...\n'Current month/day/year' exist?\nIf not, create a new folder with that name"
                        n107 = String To Path(string=w218) -> (path=w223:path)
                        n108 = String To Path(string=w219) -> (path=w221:path)
                        n109 = call <vilib>:"Check if File or Folder Exists.vi"("path"=w223) -> ("file or folder exists?"=w222:bool)  [unwired: 8 in, 2 out]
                        n110 = call <vilib>:"Check if File or Folder Exists.vi"("path"=w221) -> ("file or folder exists?"=w220:bool)  [unwired: 8 in, 2 out]
                        n111 = case shown="False" w222 {
                          tunnel: w223 -> [w225 _]
                          frame False {
                            # "create new folder"
                            n112 = Create Folder(path (use dialog)=w225) -> ()  [unwired: 2 in, 3 out]
                          }
                          frame True {
                            # "Folder exists\ndo nothing"
                          }
                        }
                        n113 = case shown="False" w220 {
                          tunnel: w221 -> [w224 _]
                          frame False {
                            # "create new folder"
                            n114 = Create Folder(path (use dialog)=w224) -> ()  [unwired: 2 in, 3 out]
                          }
                          frame True {
                            # "Folder exists\ndo nothing"
                          }
                        }
                      }
                    }
                    n115 = Concatenate Strings(w187, "\\" ("string")) -> (w194:string)
                    n116 = Concatenate Strings(w186, "\\" ("string")) -> (w189:string)
                    n117 = Format Date/Time String(time format string (%c)="%H", seconds (now)=w185) -> (date/time string=w197:string)  [unwired: 1 in]
                    n118 = Format Date/Time String(time format string (%c)="%H", seconds (now)=w185) -> (date/time string=w192:string)  [unwired: 1 in]
                    n119 = Concatenate Strings(w194, w197) -> (w157:string)
                    "File Path_Far Field (out)" <- w157
                    n120 = Concatenate Strings(w189, w192) -> (w158:string)
                    "File Path_Near Field (out)" <- w158
                    n121 = String To Path(string=w157) -> (path=w195:path)
                    n122 = String To Path(string=w158) -> (path=w190:path)
                    n123 = call <vilib>:"Check if File or Folder Exists.vi"("path"=w195) -> ("file or folder exists?"=w184:bool, "dup path"=w182:path)  [unwired: 8 in, 1 out]
                    n124 = call <vilib>:"Check if File or Folder Exists.vi"("path"=w190) -> ("file or folder exists?"=w183:bool, "dup path"=w181:path)  [unwired: 8 in, 1 out]
                    n125 = case shown="False" w184 {
                      tunnel: w182 -> [w216 _]
                      tunnel: w157 -> [w215 w217]
                      tunnel: [w215 w217] -> w155
                      frame False {
                        # "new folder"
                        n126 = Create Folder(path (use dialog)=w216) -> ()  [unwired: 2 in, 3 out]
                      }
                      frame True {
                        # "Folder exists\ndo nothing"
                      }
                    }
                    n127 = case shown="False" w183 {
                      tunnel: w181 -> [w213 _]
                      tunnel: w158 -> [w212 w214]
                      tunnel: [w212 w214] -> w156
                      frame False {
                        # "new folder"
                        n128 = Create Folder(path (use dialog)=w213) -> ()  [unwired: 2 in, 3 out]
                      }
                      frame True {
                        # "Folder exists\ndo nothing"
                      }
                    }
                    n129 = Concatenate Strings(w156, "\\Online_Raw_Data.dat" ("string")) -> (w175:string)
                    n130 = Concatenate Strings(w156, "\\Offline_Raw_Data.dat" ("string")) -> (w174:string)
                    n131 = Concatenate Strings(w155, "\\Online_Raw_Data.dat" ("string")) -> (w180:string)
                    n132 = Concatenate Strings(w155, "\\Offline_Raw_Data.dat" ("string")) -> (w179:string)
                    n133 = local read "DataOpen"() -> (w172:bool)
                    n134 = String To Path(string=w180) -> (path=w171:path)
                    n135 = String To Path(string=w179) -> (path=w170:path)
                    n136 = String To Path(string=w175) -> (path=w169:path)
                    n137 = String To Path(string=w174) -> (path=w168:path)
                    n138 = case shown="True" w172 {
                      tunnel: w171 -> [w203 w207]
                      tunnel: [w203 w207] -> w165
                      tunnel: w170 -> [w202 w206]
                      tunnel: [w202 w206] -> w164
                      tunnel: w169 -> [w201 w205]
                      tunnel: [w201 w205] -> w163
                      tunnel: [w200 w204] -> w162
                      tunnel: w168 -> [w200 w204]
                      frame False {
                        # "No files open\ndo nothing"
                      }
                      frame True {
                        # "Close open files"
                        n139 = local read "NF_Off_Ref"() -> (w209:refnum<file>)
                        n140 = local read "NF_On_Ref"() -> (w208:refnum<file>)
                        n141 = local read "FF_Off_Ref"() -> (w211:refnum<file>)
                        n142 = local read "FF_On_Ref"() -> (w210:refnum<file>)
                        n143 = Close File(refnum=w210) -> ()  [unwired: 1 in, 2 out]
                        n144 = Close File(refnum=w211) -> ()  [unwired: 1 in, 2 out]
                        n145 = Close File(refnum=w208) -> ()  [unwired: 1 in, 2 out]
                        n146 = Close File(refnum=w209) -> ()  [unwired: 1 in, 2 out]
                      }
                    }
                    n147 = Open/Create/Replace File(file path (use dialog)=w165, operation (0:open)=T7."open or create") -> (refnum out=w151:refnum<file>)  [unwired: 4 in, 2 out]
                    n148 = Open/Create/Replace File(file path (use dialog)=w164, operation (0:open)=T7."open or create") -> (refnum out=w152:refnum<file>)  [unwired: 4 in, 2 out]
                    n149 = Open/Create/Replace File(file path (use dialog)=w163, operation (0:open)=T7."open or create") -> (refnum out=w153:refnum<file>)  [unwired: 4 in, 2 out]
                    n150 = Open/Create/Replace File(file path (use dialog)=w162, operation (0:open)=T7."open or create") -> (refnum out=w154:refnum<file>)  [unwired: 4 in, 2 out]
                    n151 = Get File Size(file=w151) -> (refnum out=→"FF_On_Ref":refnum<file>, size (in bytes)=→"FF_On_Ptr":i64)  [unwired: 1 in, 1 out]
                    n152 = Get File Size(file=w152) -> (refnum out=→"FF_Off_Ref":refnum<file>, size (in bytes)=→"FF_Off_Ptr":i64)  [unwired: 1 in, 1 out]
                    n153 = Get File Size(file=w153) -> (refnum out=→"NF_On_Ref":refnum<file>, size (in bytes)=→"NF_On_Ptr":i64)  [unwired: 1 in, 1 out]
                    n154 = Get File Size(file=w154) -> (refnum out=→"NF_Off_Ref":refnum<file>, size (in bytes)=→"NF_Off_Ptr":i64)  [unwired: 1 in, 1 out]
                  }
                  frame True {
                    # "Don't need to do anything!"
                  }
                }
              }
              frame #1 {
                # "Writing and plotting retrieved\nweather parameters"
                # "Matlab script goes online and retrieves most recent press, temp, and relative humidity data \nfrom the weather station on the roof of Cobleigh"
                # "Importing the current weather conditions from the COE weather station"
                n155 = disable-structure shown="Disabled" {
                  frame Disabled {
                    n156 = script code="%try\n%s=urlread('http://www.coe.montana.edu/ee/weather/mostCurrentCSV.php');\n%amin=textscan(s,'%s %s %s %s %s %s %s %s %s %s %s %s %s');\n%data=amin{1}{2};\n%[test remain]=strtok(data,',');\n%remain=str2num(remain);\n%press=remain(3)./1000;\n%temp=remain(5);\n%RH=remain(7);\n%catch\npress=.850;\ntemp=20;\nRH=40;\n%end"() -> ()  [unwired: 1 in, 4 out]
                  }
                  frame Enabled {
                  }
                }
                "Temperature (C)" <- "Temperature (C)"
                "Pressure (mb)" <- "Pressure (mbar or hPa)"
                "Relative Humdity (%)" <- 40.0 ("Real")
              }
              frame #2 {
                # "Frame 3: Read, process, and plot online data\nFrame 4:\nFrame 5: Write the data to the folders from Frame 0 of outter sequence"
                # "Frame 0: Read the online wavelength and adjust to locking tolerance if out of range, Switch to offline DBR\nFrame 1: Read the output power from the Newport meter, calculate and plot the output pulse energy\nFrame 2: Wait 'Scalar Wait Time' for buffer to clear other wavelength data"
                # "Online"
                n157 = stacked-sequence {
                  frame #0 {
                    n158 = local read "L_Count"() -> (w235:i32)
                    n159 = Add(x=w235, y=60) -> (x+y=w233:i32)
                    n160 = Quotient & Remainder(x=w233, y=1.0) -> (x-y*floor(x/y)=w237:dbl)  [unwired: 1 out]
                    n161 = Equal To 0?(x=w237) -> (x = 0?=w236:bool)
                    n162 = case shown="True" w236 {
                      frame False {
                      }
                      frame True {
                        # "Read the online wavelength and continue adjusting the online DBR if outside the wavelength tolerance\nuntil it is within tolerance"
                        n163 = flat-sequence {
                          frame #0 {
                            # "Set the TSOA switch to\namplify the ABSORBING\nwavelength"
                            n164 = Build Array(FALSE ("Boolean")) -> (w239:bool[])
                            n165 = call-poly <vilib>:"DAQmx Write.vi"("task/channels in"=refnum<k21> "BristolWM", "data"=w239) -> ()  [unwired: 11 in, 3 out]
                          }
                          frame #1 {
                            n166 = while {
                              stop <- w242 stop-if-true
                              # "If WL difference is within tolerance, stop looping, and illuminate 'Wavelength Lock Online' indicator"
                              # "Frame 2: Decrement DBR current if above tolerance\nFrame 3: Increment DBR current if below tolerance"
                              # "Frame 0: Read the current wavelength from the wavemeter\nFrame 1: Calculate the difference between desired and actual wavelength"
                              # "Continue reading and adjusting online DBR current until within locking tolerance"
                              n167 = local read "AB_DIF"() -> (w245:dbl)
                              n168 = local read "ILX Address On"() -> (w243:dbl)
                              n169 = stacked-sequence {
                                tunnel: w243 -> [_ _ w261 w278]
                                frame #0 {
                                # "Reading the wavelength from the wavemeter"
                                n170 = flat-sequence {
                                tunnel: [w251] -> w250
                                tunnel: w250 -> [w254]
                                tunnel: [w253] -> w249
                                tunnel: w249 -> [w257]
                                frame #0 {
                                n171 = local read "Bristol In"() -> (w252:i32)
                                n172 = dll-call lib="C:/Users/H2ODial/Desktop/Shared Telescope WV DIAL Code/Libraries and VIs/CLDevIface.dll" fn="CLOpenUSBSerialDevice"("commPort"=w252) -> ("return type"=w251:i32)  [unwired: 4 in, 2 out]
                                }
                                frame #1 {
                                n173 = dll-call lib="C:/Users/H2ODial/Desktop/Shared Telescope WV DIAL Code/Libraries and VIs/CLDevIface.dll" fn="CLGetLambdaReading"("devHandle"=w254) -> ("return type"=→"Lambda On Read (nm)":dbl, "devHandle"=w253:i32)  [unwired: 3 in, 2 out]
                                }
                                frame #2 {
                                n174 = dll-call lib="C:/Users/H2ODial/Desktop/Shared Telescope WV DIAL Code/Libraries and VIs/CLDevIface.dll" fn="CLCloseDevice"("commPort"=w257) -> ("return type"=w256:i32)  [unwired: 4 in, 2 out]
                                n175 = local write "Bristol Out"(w256) -> ()
                                }
                                }
                                }
                                frame #1 {
                                # "Calculating the difference between the actual and desired online wavelength"
                                n176 = local read "Lambda On Read (nm)"() -> (w260:dbl)
                                n177 = Subtract(x=w260, y="Lambda On Set (nm)") -> (x-y=→"AB_DIF":dbl)
                                }
                                frame #2 {
                                # "If the wavelength difference is greater that 0.0002 nm, decrement the \nDBR current by 0.01 mA"
                                n178 = local read "AB_DIF"() -> (w264:dbl)
                                n179 = Greater Or Equal?(x=w264, y=0.0001) -> (x >= y?=w262:bool)
                                n180 = case shown="True" w262 {
                                tunnel: w261 -> [_ w265]
                                frame False {
                                # "Wavelength difference is not greater than 0.0002 nm, do nothing"
                                }
                                frame True {
                                n181 = stacked-sequence {
                                tunnel: w265 -> [w266 w269]
                                frame #0 {
                                # "Specifying laser channel 1,\nwhich is the online channel"
                                n182 = Number To Decimal String(number=w266) -> (decimal integer string=w267:string)  [unwired: 1 in]
                                n183 = GPIB Write(0:w267, 1:"LAS:CHAN 2") -> ()  [unwired: 3 in, 2 out]
                                }
                                frame #1 {
                                # "issuing the command"
                                # "Generating a command string\nto decrement the current"
                                # "WL difference is greater than 0.0002 nm,\ndecrement the DBR current by 0.01 mA"
                                n184 = local read "Lambda On DBR Current"() -> (w276:dbl)
                                n185 = Subtract(x=w276, y=0.01) -> (x-y=w270:dbl)
                                n186 = local write "Lambda On DBR Current"(w270) -> ()
                                n187 = Format Into String(format string="%.4f" ("Format String"), w270) -> (resulting string=w273:string)  [unwired: 2 in, 1 out]
                                n188 = Concatenate Strings("LAS:LDI ", w273) -> (w272:string)
                                n189 = Number To Decimal String(number=w269) -> (decimal integer string=w271:string)  [unwired: 1 in]
                                n190 = GPIB Write(0:w271, 1:w272) -> ()  [unwired: 3 in, 2 out]
                                }
                                }
                                }
                                }
                                }
                                frame #3 {
                                # "If WL difference is < 0.0002 nm, increment the DBR current"
                                n191 = local read "AB_DIF"() -> (w281:dbl)
                                n192 = Less Or Equal?(x=w281, y=-0.0001) -> (x <= y?=w279:bool)
                                n193 = case shown="True" w279 {
                                tunnel: w278 -> [_ w282]
                                frame False {
                                # "WL difference is no <= to -0.0002 nm, do nothing"
                                }
                                frame True {
                                n194 = stacked-sequence {
                                tunnel: w282 -> [w284 w286]
                                frame #0 {
                                # "Specifying laser channel 1,\nwhich is the online channel"
                                n195 = Number To Decimal String(number=w284) -> (decimal integer string=w283:string)  [unwired: 1 in]
                                n196 = GPIB Write(0:w283, 1:"LAS:CHAN 2") -> ()  [unwired: 3 in, 2 out]
                                }
                                frame #1 {
                                # "issuing the command"
                                # "Generating a command \nstring to increment the current"
                                # "WL difference is < -0.0002,\nincrement the DBR current by 0.01 mA"
                                n197 = local read "Lambda On DBR Current"() -> (w293:dbl)
                                n198 = Add(x=w293, y=0.01) -> (x+y=w288:dbl)
                                n199 = local write "Lambda On DBR Current"(w288) -> ()
                                n200 = Format Into String(format string="%.4f" ("Format String"), w288) -> (resulting string=w290:string)  [unwired: 2 in, 1 out]
                                n201 = Concatenate Strings("LAS:LDI ", w290) -> (w289:string)
                                n202 = Number To Decimal String(number=w286) -> (decimal integer string=w287:string)  [unwired: 1 in]
                                n203 = GPIB Write(0:w287, 1:w289) -> ()  [unwired: 3 in, 2 out]
                                }
                                }
                                }
                                }
                                }
                              }
                              n204 = Greater?(x=w245, y=-0.00011) -> (0:w247:bool)
                              n205 = Less?(x=w245, y=0.00011) -> (x < y?=w246:bool)
                              n206 = And(x=w247, y=w246) -> (x .and. y?=w242:bool)
                              "Wavelength Lock Online" <- w242
                            }
                          }
                          frame #2 {
                          }
                        }
                      }
                    }
                  }
                  frame #1 {
                    # "Converting to pulse energy, assumes 5 percent pickoff"
                    # "Reading the Newport Power meter"
                    # "Reading the output power of the laser transmitter from the Newport power meter, once read, convert to corresponding pulse energy and plot"
                    n207 = local read "Newport Device Key"() -> (w299:string)
                    n208 = local read "NewportRef"() -> (w295:refnum<k24>)
                    n209 = disable-structure shown="Disabled" {
                      frame Disabled {
                        # "Plotting the online and offling pulse energies"
                        n210 = local read "Online Pulse Energy"() -> (w310:dbl)
                        n211 = local read "Offline Pulse Energy"() -> (w309:dbl)
                        n212 = Bundle("Online Pulse Energy"=w310, "Offline Pulse Energy"=w309) -> (→"Pulse Energy (Micro Joule)":T9)  [unwired: 1 in]
                      }
                      frame Enabled {
                      }
                    }
                    n213 = Number To Decimal String(number="SampleSize") -> (decimal integer string=w297:string)  [unwired: 1 in]
                    n214 = invoke class="PowerMeterCommands" method="PerformDAQ"(reference=w295, "deviceKey"=w299, "interval"="1", "sampleSize"=w297) -> ("PerformDAQ"=w300:dbl[])  [unwired: 2 in, 5 out]
                    n215 = call-poly <vilib>:"Mean.vi"("X"=w300) -> ("mean"=w298:dbl)  [unwired: 1 out]
                    n216 = Multiply(x=w298, y=1000.0) -> (x*y=w306:dbl)
                    n217 = Divide(x=w306, y=0.05) -> (x/y=w304:dbl)
                    n218 = Divide(x=w304, y=7.0) -> (x/y=→"Online Pulse Energy":dbl)
                  }
                  frame #2 {
                    # "Wait 'Scalar Wait Time' for the next available batch of scalar card data"
                    n219 = local read "AMCS_Profile"() -> (w311:i32)
                    n220 = disable-structure shown="Disabled" {
                      frame Disabled {
                        # "Waiting 'Scalar Wait Time'"
                        n221 = Wait (ms)(milliseconds to wait="Scalar Wait Time") -> ()  [unwired: 1 out]
                      }
                      frame Enabled {
                      }
                    }
                    n222 = while {
                      tunnel: [w318] -> w312
                      tunnel: [w314] -> _
                      tunnel: w311 -> [w314]
                      stop <- w316 stop-if-true
                      n223 = global read "AMCS_Data.vi" "AMCS_Profile"() -> (w318:i32)
                      n224 = Wait (ms)(milliseconds to wait=u32 10) -> ()  [unwired: 1 out]
                      n225 = Equal?(x=w318, y=w314) -> (x = y?=w317:bool)
                      n226 = case shown="False" w317 {
                        tunnel: [TRUE FALSE] -> w316
                        frame False {
                        }
                        frame True {
                        }
                      }
                    }
                    "AMCS_Profile" <- w312
                  }
                  frame #3 {
                    # "convert time per range bin to meters\nand calculate smoothed bins using\nsmoothing range"
                    # "Plotting online cross section and smoothed online data"
                    # "Calculate the bin by bin mean of the data"
                    # "Collect 'Integration Period (Seconds)' number\nof scalar data"
                    # "Reading, processing, and plotting the online data"
                    n227 = local read "Data Reads (number of loops)"() -> (w346:i32)
                    n228 = for {
                      N: w346 -> [_]
                      tunnel: [w367] -> w358 mode=indexing
                      tunnel: [w366] -> w321 mode=indexing
                      # "Scalar Data is retrieved from Global \nVariable that scaler.vi is writing to,"
                      n229 = global read "AMCS_Data.vi" "AMCS_Data"() -> (w370:u16[][])
                      n230 = disable-structure shown="Disabled" {
                        frame Disabled {
                          n231 = global read "Scalar_Data_3.vi" "Scalar Data 3"() -> ()  [unwired: 1 out]
                          n232 = global read "Scalar_Data.vi" "Scalar Data"() -> ()  [unwired: 1 out]
                        }
                        frame Enabled {
                        }
                      }
                      n233 = Index Array(array=w370, index (row) #1=0 ("index (row)"), index (row) #2=2 ("index (row)")) -> (element #1=w367:u16[], element #2=w366:u16[])  [unwired: 2 in]
                    }
                    n234 = Transpose 2D Array(2D array=w358) -> (transposed array=w362:u16[][])
                    n235 = Transpose 2D Array(2D array=w321) -> (transposed array=w344:u16[][])
                    n236 = for {
                      tunnel: w362 -> [w372] mode=indexing
                      tunnel: [w371] -> w363 mode=indexing
                      n237 = call-poly <vilib>:"Mean.vi"("X"=w372) -> ("mean"=w371:dbl)  [unwired: 1 out]
                    }
                    n238 = for {
                      tunnel: w344 -> [w365] mode=indexing
                      tunnel: [w364] -> w345 mode=indexing
                      n239 = call-poly <vilib>:"Mean.vi"("X"=w365) -> ("mean"=w364:dbl)  [unwired: 1 out]
                    }
                    n240 = local read "bins"() -> (w338:u32)
                    n241 = Array Subset(array=w363, index=1 ("dimension size"), length=w338) -> (w350:dbl[])
                    n242 = Array Subset(array=w345, index=1 ("dimension size"), length=w338) -> (w342:dbl[])
                    n243 = local read "background length"() -> (w328:i32)
                    n244 = local read "background start"() -> (w329:u32)
                    n245 = Array Size(array=w350) -> (size(s)=w347:i32)
                    n246 = Array Size(array=w342) -> (size(s)=w339:i32)
                    n247 = Initialize Array(1.0 ("element"), w347) -> (w349:dbl[])
                    n248 = Initialize Array(1.0 ("element"), w339) -> (w341:dbl[])
                    n249 = Multiply(x=w350, y=w349) -> (x*y=w351:dbl[])
                    "On-Line Bin Readings" <- w351
                    n250 = Multiply(x=w342, y=w341) -> (x*y=w332:dbl[])
                    "On-Line Bin Readings 2" <- w332
                    n251 = local read "Total DIAL Integration Time (Minutes)"() -> (w354:i32)
                    n252 = local read "Time Resolution Per Bin(ns)"() -> (w324:u32)
                    n253 = Array Subset(array=w351, index=w329, length=w328) -> (w360:dbl[])
                    n254 = Array Subset(array=w332, index=w329, length=w328) -> (w334:dbl[])
                    n255 = call-poly <vilib>:"Mean.vi"("X"=w360) -> ("mean"=w359:dbl)  [unwired: 1 out]
                    n256 = call-poly <vilib>:"Mean.vi"("X"=w334) -> ("mean"=w335:dbl)  [unwired: 1 out]
                    n257 = Divide(x=w354, y=w346) -> (x/y=w352:dbl)
                    n258 = local read "Index"() -> (w333:i32)
                    n259 = Subtract(x=w351, y=w359) -> (x-y=w356:dbl[])
                    n260 = Subtract(x=w332, y=w335) -> (x-y=w336:dbl[])
                    n261 = To Double Precision Float(number=w324) -> (double precision float=w325:dbl)
                    n262 = Multiply(x=w352, y=60.0) -> (x*y=w330:dbl)
                    n263 = Multiply(x=w325, y=0.15) -> (x*y=w327:dbl)
                    n264 = call "Ring Buffer Online Far.vi"("Index"=w333, "Profiles to Average"=w330, "Input Array"=w356) -> ("AvgArray"=w355:dbl[])  [unwired: 7 in, 1 out]
                    n265 = call "Ring Buffer Online Near.vi"("Index"=w333, "Profiles to Average"=w330, "Input Array"=w336) -> ("AvgArray"=w337:dbl[])  [unwired: 7 in, 1 out]
                    n266 = Divide(x="Smoothing Range", y=w327) -> (x/y=w322:dbl)
                    "Smoothed Bins" <- w322
                    n267 = call "Smooth Arrray.vi"("smooth size"=w322, "Raw Array"=w355) -> ("Smoothed Array"=→"On-Line  Smoothed":dbl[])  [unwired: 9 in]
                    n268 = call "Smooth Arrray.vi"("smooth size"=w322, "Raw Array"=w337) -> ("Smoothed Array"=→"On-Line Smoothed 2":dbl[])  [unwired: 9 in]
                    n269 = disable-structure shown="Disabled" {
                      frame Disabled {
                        n270 = script code="format long;\ncounts=sum(Online);\nif counts >=0.5e6\ntime=time;\nelse\ntime=time\nend"() -> ()  [unwired: 3 in, 2 out]
                      }
                      frame Enabled {
                      }
                    }
                  }
                  frame #4 {
                    # "Toggling the Agiltron switch to the offline DBR seed laser"
                    n271 = disable-structure shown="Disabled" {
                      frame Disabled {
                        n272 = flat-sequence {
                          frame #0 {
                            # "Second one"
                            # "Command the switch to switch to position 2\ncorresponding to the offline DBR"
                            # "Hex string command \ncorrespond to offline"
                            n273 = VISA Write(VISA resource name="Switch Comm Port", write buffer="\u0001\u0012\u0000\u0001") -> ()  [unwired: 1 in, 3 out]
                          }
                        }
                      }
                      frame Enabled {
                      }
                    }
                  }
                  frame #5 {
                    # "Save the recently collected online data if 'Save Data?' is true"
                    n274 = case shown="True" "Save Data?" {
                      frame False {
                        # "'Save Data?' is false, do nothing"
                      }
                      frame True {
                        # "'Save Data?' is true, save onfline data to the Data Disk"
                        # "Write only one copy of data at this time"
                        # "Retrieve Julian Date"
                        n275 = local read "Lambda On DBR Current"() -> (w400:dbl)
                        n276 = local read "Lambda On Read (nm)"() -> (w401:dbl)
                        n277 = local read "On-Line Bin Readings 2"() -> (w395:dbl[])
                        n278 = local read "Relative Humdity (%)"() -> (w396:dbl)
                        n279 = local read "On-Line Bin Readings"() -> (w403:dbl[])
                        n280 = local read "Online Pulse Energy"() -> (w399:dbl)
                        n281 = local read "Temperature (C)"() -> (w398:dbl)
                        n282 = local read "Pressure (mb)"() -> (w397:dbl)
                        n283 = call "Julian_Date_2.vi"() -> ("Julian Date"=w402:dbl)  [unwired: 11 in]
                        n284 = Build Array (concatenate)(w402, w401, w400, w399, w398, w397, w396, w403) -> (w390:dbl[])
                        n285 = Build Array (concatenate)(w402, w401, w400, w399, w398, w397, w396, w395) -> (w380:dbl[])
                        n286 = local write "DataOpen"(TRUE ("DataOpen")) -> ()
                        n287 = local read "NF_On_Ref"() -> (w378:refnum<file>)
                        n288 = local read "FF_On_Ref"() -> (w394:refnum<file>)
                        n289 = local read "NF_On_Ptr"() -> (w379:i64)
                        n290 = local read "FF_On_Ptr"() -> (w393:i64)
                        n291 = Set File Position(offset (in bytes) (0)=w393, refnum=w394) -> (refnum out=w391:refnum<file>, error out=w388:errorcluster)  [unwired: 2 in]
                        n292 = Set File Position(offset (in bytes) (0)=w379, refnum=w378) -> (refnum out=w384:refnum<file>, error out=w382:errorcluster)  [unwired: 2 in]
                        n293 = Write to Binary File(file (use dialog)=w384, data=w380, error in=w382, 5:FALSE ("prepend array or string size? (T)")) -> (refnum out=w383:refnum<file>, error out=w381:errorcluster)  [unwired: 2 in, 1 out]
                        n294 = Write to Binary File(file (use dialog)=w391, data=w390, error in=w388, 5:FALSE ("prepend array or string size? (T)")) -> (refnum out=w389:refnum<file>, error out=w387:errorcluster)  [unwired: 2 in, 1 out]
                        n295 = Get File Position(4:w381, 7:w383) -> (2:w377:i64)  [unwired: 2 out]
                        n296 = Get File Position(4:w387, 7:w389) -> (2:w386:i64)  [unwired: 2 out]
                        n297 = local write "NF_On_Ptr"(w377) -> ()
                        n298 = local write "FF_On_Ptr"(w386) -> ()
                      }
                    }
                  }
                }
              }
              frame #3 {
                # "Frame 3: Read offline data, calculate aerosol data, and plot offline and normalized relative backscatter\nFrame 4:\nFrame 5: Save the offline data and related information"
                # "Frame 0: Read the offline wavelength and lock if necessary, Switch to online DBR\nFrame 1: Read the output power from the Newport power meter\nFrame 2: Wait 'Scalar Wait Time' for buffers to clear of online contiminated data"
                # "offline"
                n299 = stacked-sequence {
                  frame #0 {
                    # "Every 60 data collection cycles, read the offline DBR wavelength, and if outside of wavelength tolerance, adjust DBR current until within tolerance"
                    n300 = local read "L_Count"() -> (w405:i32)
                    n301 = Quotient & Remainder(x=w405, y=60.0) -> (x-y*floor(x/y)=w406:dbl)  [unwired: 1 out]
                    n302 = Equal To 0?(x=w406) -> (x = 0?=w404:bool)
                    n303 = case shown="True" w404 {
                      frame False {
                      }
                      frame True {
                        n304 = flat-sequence {
                          frame #0 {
                            # "Set the TSOA switch to\namplify the non ABSORBING\nwavelength"
                            n305 = Build Array(TRUE ("Boolean")) -> (w409:bool[])
                            n306 = Wait (ms)(milliseconds to wait=u32 3200) -> ()  [unwired: 1 out]
                            n307 = call-poly <vilib>:"DAQmx Write.vi"("task/channels in"=refnum<k21> "BristolWM", "data"=w409) -> ()  [unwired: 11 in, 3 out]
                          }
                          frame #1 {
                            n308 = while {
                              stop <- w412 stop-if-true
                              # "If WL difference is within tolerance, stop looping, and illuminate 'Wavelength Lock Offline' indicator"
                              # "Frame 2: Decrement DBR current if above tolerance\nFrame 3: Increment DBR current if below tolerance"
                              # "Frame 0: Read the current wavelength from the wavemeter\nFrame 1: Calculate the difference between desired and actual wavelength"
                              # "Continue reading and adjusting offline DBR current until within locking tolerance"
                              n309 = local read "NONAB_DIF"() -> (w415:dbl)
                              n310 = local read "ILX Address Off"() -> (w413:dbl)
                              n311 = stacked-sequence {
                                tunnel: w413 -> [_ _ w431 w448]
                                frame #0 {
                                # "Reading the wavelength from the wavemeter"
                                n312 = flat-sequence {
                                tunnel: [w421] -> w420
                                tunnel: w420 -> [w424]
                                tunnel: [w423] -> w419
                                tunnel: w419 -> [w427]
                                frame #0 {
                                n313 = local read "Bristol In"() -> (w422:i32)
                                n314 = dll-call lib="C:/Users/H2ODial/Desktop/Shared Telescope WV DIAL Code/Libraries and VIs/CLDevIface.dll" fn="CLOpenUSBSerialDevice"("commPort"=w422) -> ("return type"=w421:i32)  [unwired: 4 in, 2 out]
                                }
                                frame #1 {
                                n315 = dll-call lib="C:/Users/H2ODial/Desktop/Shared Telescope WV DIAL Code/Libraries and VIs/CLDevIface.dll" fn="CLGetLambdaReading"("devHandle"=w424) -> ("return type"=→"Lambda Off Read (nm)":dbl, "devHandle"=w423:i32)  [unwired: 3 in, 2 out]
                                }
                                frame #2 {
                                n316 = dll-call lib="C:/Users/H2ODial/Desktop/Shared Telescope WV DIAL Code/Libraries and VIs/CLDevIface.dll" fn="CLCloseDevice"("commPort"=w427) -> ("return type"=w426:i32)  [unwired: 4 in, 2 out]
                                n317 = local write "Bristol Out"(w426) -> ()
                                }
                                }
                                }
                                frame #1 {
                                # "Calculating the difference between the actual and desired online wavelength"
                                n318 = local read "Lambda Off Read (nm)"() -> (w430:dbl)
                                n319 = Subtract(x=w430, y="Lambda Off Set (nm)") -> (x-y=→"NONAB_DIF":dbl)
                                }
                                frame #2 {
                                # "If the wavelength difference is greater that 0.0002 nm, decrement the \nDBR current by 0.01 mA"
                                n320 = local read "NONAB_DIF"() -> (w434:dbl)
                                n321 = Greater Or Equal?(x=w434, y=0.0001) -> (x >= y?=w432:bool)
                                n322 = case shown="True" w432 {
                                tunnel: w431 -> [_ w435]
                                frame False {
                                # "Wavelength difference is not greater than 0.0002 nm, do nothing"
                                }
                                frame True {
                                n323 = stacked-sequence {
                                tunnel: w435 -> [w436 w439]
                                frame #0 {
                                # "Specifying laser channel 1,\nwhich is the online channel"
                                n324 = Number To Decimal String(number=w436) -> (decimal integer string=w437:string)  [unwired: 1 in]
                                n325 = GPIB Write(0:w437, 1:"LAS:CHAN 2") -> ()  [unwired: 3 in, 2 out]
                                }
                                frame #1 {
                                # "issuing the command"
                                # "Generating a command string\nto decrement the current"
                                # "WL difference is greater than 0.0002 nm,\ndecrement the DBR current by 0.01 mA"
                                n326 = local read "Lambda Off DBR Current"() -> (w446:dbl)
                                n327 = Subtract(x=w446, y=0.01) -> (x-y=w440:dbl)
                                n328 = local write "Lambda Off DBR Current"(w440) -> ()
                                n329 = Format Into String(format string="%.4f" ("Format String"), w440) -> (resulting string=w443:string)  [unwired: 2 in, 1 out]
                                n330 = Concatenate Strings("LAS:LDI ", w443) -> (w442:string)
                                n331 = Number To Decimal String(number=w439) -> (decimal integer string=w441:string)  [unwired: 1 in]
                                n332 = GPIB Write(0:w441, 1:w442) -> ()  [unwired: 3 in, 2 out]
                                }
                                }
                                }
                                }
                                }
                                frame #3 {
                                # "If WL difference is < 0.0002 nm, increment the DBR current"
                                n333 = local read "NONAB_DIF"() -> (w451:dbl)
                                n334 = Less Or Equal?(x=w451, y=-0.0001) -> (x <= y?=w449:bool)
                                n335 = case shown="True" w449 {
                                tunnel: w448 -> [_ w452]
                                frame False {
                                # "WL difference is no <= to -0.0002 nm, do nothing"
                                }
                                frame True {
                                n336 = stacked-sequence {
                                tunnel: w452 -> [w454 w456]
                                frame #0 {
                                # "Specifying laser channel 1,\nwhich is the online channel"
                                n337 = Number To Decimal String(number=w454) -> (decimal integer string=w453:string)  [unwired: 1 in]
                                n338 = GPIB Write(0:w453, 1:"LAS:CHAN 2") -> ()  [unwired: 3 in, 2 out]
                                }
                                frame #1 {
                                # "issuing the command"
                                # "Generating a command \nstring to increment the current"
                                # "WL difference is < -0.0002,\nincrement the DBR current by 0.01 mA"
                                n339 = local read "Lambda Off DBR Current"() -> (w463:dbl)
                                n340 = Add(x=w463, y=0.01) -> (x+y=w458:dbl)
                                n341 = local write "Lambda Off DBR Current"(w458) -> ()
                                n342 = Format Into String(format string="%.4f" ("Format String"), w458) -> (resulting string=w460:string)  [unwired: 2 in, 1 out]
                                n343 = Concatenate Strings("LAS:LDI ", w460) -> (w459:string)
                                n344 = Number To Decimal String(number=w456) -> (decimal integer string=w457:string)  [unwired: 1 in]
                                n345 = GPIB Write(0:w457, 1:w459) -> ()  [unwired: 3 in, 2 out]
                                }
                                }
                                }
                                }
                                }
                              }
                              n346 = Greater?(x=w415, y=-0.00011) -> (0:w417:bool)
                              n347 = Less?(x=w415, y=0.00011) -> (x < y?=w416:bool)
                              n348 = And(x=w417, y=w416) -> (x .and. y?=w412:bool)
                              "Wavelength Lock Offline" <- w412
                            }
                          }
                          frame #2 {
                            # "Set the TSOA switch to\namplify the ABSORBING\nwavelength"
                            n349 = Build Array(FALSE ("Boolean")) -> (w465:bool[])
                            n350 = call-poly <vilib>:"DAQmx Write.vi"("task/channels in"=refnum<k21> "BristolWM", "data"=w465) -> ()  [unwired: 11 in, 3 out]
                          }
                        }
                      }
                    }
                  }
                  frame #1 {
                    # "Reading the power meter"
                    # "Updating the pulse energy plot"
                    # "Converting to pulse energy"
                    # "Reading the offline output power, converting to pulse energy,  and updating the Pulse energy plot"
                    n351 = local read "SampleSize"() -> (w470:i32)
                    n352 = local read "Newport Device Key"() -> (w471:string)
                    n353 = local read "Online Pulse Energy"() -> (w477:dbl)
                    n354 = local read "Offline Pulse Energy"() -> (w476:dbl)
                    n355 = local read "NewportRef"() -> (w468:refnum<k24>)
                    n356 = Number To Decimal String(number=w470) -> (decimal integer string=w472:string)  [unwired: 1 in]
                    n357 = invoke class="PowerMeterCommands" method="PerformDAQ"(reference=w468, "deviceKey"=w471, "interval"="1", "sampleSize"=w472) -> ("PerformDAQ"=w473:dbl[])  [unwired: 2 in, 5 out]
                    n358 = Bundle("Online Pulse Energy"=w477, "Offline Pulse Energy"=w476) -> (w475:T9)  [unwired: 1 in]
                    n359 = local write "Pulse Energy (Micro Joule)"(w475) -> ()
                    n360 = call-poly <vilib>:"Mean.vi"("X"=w473) -> ("mean"=w469:dbl)  [unwired: 1 out]
                    n361 = Multiply(x=w469, y=1000.0) -> (x*y=w482:dbl)
                    n362 = Divide(x=w482, y=0.05) -> (x/y=w480:dbl)
                    n363 = Divide(x=w480, y=7.0) -> (x/y=→"Offline Pulse Energy":dbl)
                  }
                  frame #2 {
                    # "Wait 'Scalar Wait Time' for buffers to clear of online contiminated offline data"
                    n364 = disable-structure shown="Disabled" {
                      frame Disabled {
                        # "Wait 'Scalar Wait Time'"
                        n365 = local read "Scalar Wait Time"() -> (w484:u32)
                        n366 = Wait (ms)(milliseconds to wait=w484) -> ()  [unwired: 1 out]
                      }
                      frame Enabled {
                      }
                    }
                  }
                  frame #3 {
                    w518 = 1 ("dimension size")
                    w522 = 1
                    # "Read in latest scalar card data from \n'Scalar Data' global variable that \nscaler.vi is writing to, then wait 1 sec\nfor next batch of data"
                    # "Plotting the normalized relative \nbackscatter"
                    # "Calculating the normalized relative backscatter"
                    # "Calculating/Plotting smoothed data,\ncross sections etc."
                    # "Pick off data with\nout header"
                    # "Calculate mean bin by bin mean"
                    # "Reading in 'Integration Period (Seconds)' of data"
                    # "Read the offline data from the scalar card, perform smoothing, calculate normalized relative backscatter, and plot"
                    # "File path in MATLAB script is of old dial is:\nF:\\Micropulse DIAL\\Micropulse DIAL Matlab\\\nFinal Overlap Function.mat')];"
                    # "Collects Data From Card,\nSends It To The Chart,\nAnd Saves A Copy As A\nFile If Option Selected On\nFront Panel"
                    n367 = for {
                      N: "Data Reads (number of loops)" -> [_]
                      tunnel: [w554] -> w486 mode=indexing
                      tunnel: [w553] -> w485 mode=indexing
                      n368 = global read "AMCS_Data.vi" "AMCS_Data"() -> (w555:u16[][])
                      n369 = disable-structure shown="Disabled" {
                        frame Disabled {
                          n370 = global read "Scalar_Data_4.vi" "Scalar Data 4"() -> ()  [unwired: 1 out]
                          n371 = global read "Scalar_Data_2.vi" "Scalar Data 2"() -> ()  [unwired: 1 out]
                        }
                        frame Enabled {
                        }
                      }
                      n372 = Index Array(array=w555, index (row) #1=1 ("index (row)"), index (row) #2=3 ("index (row)")) -> (element #1=w554:u16[], element #2=w553:u16[])  [unwired: 2 in]
                    }
                    n373 = local read "Total DIAL Integration Time (Minutes)"() -> (w543:i32)
                    n374 = Divide(x=w543, y="Data Reads (number of loops)") -> (x/y=w541:dbl)
                    n375 = local read "Total Aerosol Integration Time (Minutes)"() -> (w545:dbl)
                    n376 = local read "background length"() -> (w490:i32)
                    n377 = Multiply(x=w541, y=60.0) -> (x*y=w528:dbl)
                    n378 = local read "background start"() -> (w491:u32)
                    n379 = Transpose 2D Array(2D array=w486) -> (transposed array=w551:u16[][])
                    n380 = Transpose 2D Array(2D array=w485) -> (transposed array=w534:u16[][])
                    n381 = Divide(x=w545, y="Data Reads (number of loops)") -> (x/y=w546:dbl)
                    n382 = for {
                      tunnel: w551 -> [w561] mode=indexing
                      tunnel: [w560] -> w552 mode=indexing
                      tunnel: w534 -> [w559] mode=indexing
                      tunnel: [w558] -> _ mode=indexing
                      tunnel: [w558] -> w531 mode=indexing
                      n383 = call-poly <vilib>:"Mean.vi"("X"=w561) -> ("mean"=w560:dbl)  [unwired: 1 out]
                      n384 = call-poly <vilib>:"Mean.vi"("X"=w559) -> ("mean"=w558:dbl)  [unwired: 1 out]
                    }
                    n385 = local read "bins"() -> (w519:u32)
                    n386 = Multiply(x=w546, y=60.0) -> (x*y=w509:dbl)
                    n387 = Array Subset(array=w531, index=w518, length=w519) -> (w532:dbl[])
                    "Off-Line Bin Readings 2" <- w532
                    n388 = Array Subset(array=w552, index=w518, length=w519) -> (w530:dbl[])
                    "Off-Line  Bin Readings" <- w530
                    n389 = Array Subset(array=w532, index=w491, length=w490) -> (w533:dbl[])
                    n390 = Array Subset(array=w530, index=w491, length=w490) -> (w550:dbl[])
                    n391 = local read "Smoothed Bins"() -> (w487:dbl)
                    n392 = call-poly <vilib>:"Mean.vi"("X"=w533) -> ("mean"=w497:dbl)  [unwired: 1 out]
                    n393 = call-poly <vilib>:"Mean.vi"("X"=w550) -> ("mean"=w498:dbl)  [unwired: 1 out]
                    n394 = local read "Index"() -> (w508:i32)
                    n395 = Subtract(x=w532, y=w497) -> (x-y=w510:dbl[])
                    n396 = Subtract(x=w530, y=w498) -> (x-y=w526:dbl[])
                    n397 = call "Ring Buffer Offline Far.vi"("Index"=w508, "Profiles to Average"=w528, "Input Array"=w526) -> ("AvgArray"=w548:dbl[], "RingBufferOut"=→"RingBuffer offline far":dbl[][])  [unwired: 7 in]
                    n398 = call "Ring Buffer Aerosol Far.vi"("Index"=w508, "Profiles to Average"=w509, "Input Array"=w526) -> ("AvgArray"=w544:dbl[], "RingBufferOut"=→"RingBuffer aerosol far":dbl[][])  [unwired: 7 in]
                    n399 = call "Ring Buffer Offline Near.vi"("Index"=w508, "Profiles to Average"=w528, "Input Array"=w510) -> ("AvgArray"=w529:dbl[], "RingBufferOut"=→"RingBuffer offline near":dbl[][])  [unwired: 7 in]
                    n400 = call "Ring Buffer Aerosol Near.vi"("Index"=w508, "Profiles to Average"=w509, "Input Array"=w510) -> ("AvgArray"=w506:dbl[], "RingBufferOut"=→"RingBuffer aerosol near":dbl[][])  [unwired: 7 in]
                    n401 = Reshape Array(w526, w518, w519) -> (→"raw counts":dbl[][])
                    n402 = Reshape Array(w510, w518, w519) -> (→"raw counts near":dbl[][])
                    n403 = call "Smooth Arrray.vi"("smooth size"=w487, "Raw Array"=w548) -> ("Smoothed Array"=→"Off-Line Smoothed":dbl[])  [unwired: 9 in]
                    n404 = call "Smooth Arrray.vi"("smooth size"=w487, "Raw Array"=w544) -> ("Smoothed Array"=w517:dbl[])  [unwired: 9 in]
                    "Aerosol Smoothed" <- w517
                    n405 = call "Smooth Arrray.vi"("smooth size"=w487, "Raw Array"=w529) -> ("Smoothed Array"=→"Off-Line Smoothed 2":dbl[])  [unwired: 9 in]
                    n406 = call "Smooth Arrray.vi"("smooth size"=w487, "Raw Array"=w506) -> ("Smoothed Array"=w489:dbl[])  [unwired: 9 in]
                    "Aerosol Smoothed 2" <- w489
                    n407 = local read "Number of Accumulates"() -> (w493:u32)
                    n408 = local read "Temperature (C)"() -> (w540:dbl)
                    n409 = local read "Pressure (mb)"() -> (w539:dbl)
                    n410 = script code="%accum_num=10000;     % scaler card setting number of accumulations\nt_bin = 500e-9                 % scaler card setting time per bin\n%t_d = 37.3e-9;                % APD dead time from spec sheet\n\n% conversion from accumulated counts to count rate  (c/s)\nc_convert = 1./t_bin./accum_num;\nCR_far = p_raw_far.*c_convert;\nCR_near = p_raw_near.*c_convert;\nCR_total_far = (p_raw_far+b_far).*c_convert;\nCR_total_near = (p_raw_near+b_near).*c_convert;\nb_CR_far =b_far.*c_convert;\nb_CR_near =b_near.*c_convert;\n\n% create a range array\nsize_p =  size(p_raw_far,2);\nr = (75:75:size_p*75)./1e3; \n    \n%APD correction factor\n D_far = 1./(1-(t_d*CR_total_far));\n D_near = 1./(1-(t_d*CR_total_near));\n\n %Calculating normalize relative backscatter profile\n nrb_far = CR_far.*D_far.*r.^2./E.*1e-6;\n nrb_near = CR_near.*D_near.*r.^2./E.*1e-6;"("E"=6.0 ("Real"), "temp"=w540, "press"=w539, "p_raw_far"=w517, "b_far"=w498, "b_near"=w497, "p_raw_near"=w489, "accum_num"=w493, "t_d"="dead time") -> ("nrb_far"=w512:cdb[], "D_far"=w503:dbl[], "nrb_near"=w511:cdb[], "D_near"=w502:dbl[], "b_CR_far"=w495:dbl, "b_CR_near"=w494:dbl)  [unwired: 1 in, 1 out]
                    n411 = local read "bins"() -> (w521:u32)
                    n412 = local read "Altitude Array (km)"() -> (w514:dbl[])
                    n413 = Bundle(w495, w494) -> (→"?":cluster{dbl, dbl})  [unwired: 1 in]
                    n414 = Build Array(w512, w511) -> (w516:cdb[][])
                    n415 = Build Array(w503, w502) -> (w501:dbl[][])
                    n416 = Reshape Array(w511, w522, w521) -> (→"NRB 2":cdb[][])
                    n417 = Reshape Array(w512, w522, w521) -> (→"NRB":cdb[][])
                    n418 = Build Array(w514, w514) -> (w513:dbl[][])
                    n419 = call "Convert to Dynamic Data7"("2D Array"=w501) -> ("Dynamic Data Type"=w500:dynamicdata)  [unwired: 3 in]
                    n420 = call "Convert to Dynamic Data3"("2D Array"=w516) -> ("Dynamic Data Type"=w515:dynamicdata)  [unwired: 3 in]
                    n421 = call "Convert to Dynamic Data4"("2D Array"=w513) -> ("Dynamic Data Type"=w504:dynamicdata)  [unwired: 3 in]
                    n422 = call "Build XY Graph2"("Y Input"=w504, "X Input"=w515) -> ("XY Graph"=→"NRB plot":cluster{"Y":dbl[], "Y":dbl[]}[])  [unwired: 3 in, 6 out]
                    n423 = call "Build XY Graph4"("Y Input"=w504, "X Input"=w500) -> ("XY Graph"=→"Correction":cluster{"Y":dbl[], "Y":dbl[]}[])  [unwired: 3 in, 6 out]
                  }
                  frame #4 {
                    # "REPLACE WITH NEW AGILTRON TASK!"
                    # "Toggle Agiltron switch to online DBR"
                    n424 = disable-structure shown="Disabled" {
                      frame Disabled {
                        # "ABSORBING"
                        n425 = flat-sequence {
                          frame #0 {
                            # "Third one"
                            # "Command the switch to switch to position 1\ncorresponding to the online DBR"
                            # "Hex string command \ncorrespond to online"
                            n426 = local read "Switch Comm Port"() -> (w565:refnum<visa-resource-name>)
                            n427 = VISA Write(VISA resource name=w565, write buffer="\u0001\u0012\u0000\u0002") -> ()  [unwired: 1 in, 3 out]
                          }
                        }
                        n428 = Build Array(FALSE ("Boolean")) -> (w564:bool[])
                        n429 = call-poly <vilib>:"DAQmx Write.vi"("task/channels in"=refnum<k21> "AgiltronSwitch", "data"=w564) -> ()  [unwired: 11 in, 3 out]
                      }
                      frame Enabled {
                      }
                    }
                  }
                  frame #5 {
                    # "If 'Save Data?' is true, save all relavant offline info"
                    n430 = local read "Save Data?"() -> (w567:bool)
                    n431 = case shown="True" w567 {
                      frame False {
                        # "'Save Data?' is false, do nothing"
                      }
                      frame True {
                        # "Write only one data file at this time"
                        # "Retrive Julian Date"
                        # "'Save Data?' is true, save offline data to the Data Disk"
                        n432 = local read "Lambda Off DBR Current"() -> (w589:dbl)
                        n433 = local read "Off-Line Bin Readings 2"() -> (w586:dbl[])
                        n434 = local read "Lambda Off Read (nm)"() -> (w588:dbl)
                        n435 = local read "Off-Line  Bin Readings"() -> (w594:dbl[])
                        n436 = local read "Relative Humdity (%)"() -> (w593:dbl)
                        n437 = local read "Offline Pulse Energy"() -> (w590:dbl)
                        n438 = local read "Temperature (C)"() -> (w591:dbl)
                        n439 = local read "Pressure (mb)"() -> (w592:dbl)
                        n440 = call "Julian_Date_2.vi"() -> ("Julian Date"=w587:dbl)  [unwired: 11 in]
                        n441 = Build Array (concatenate)(w587, w588, w589, w590, w591, w592, w593, w594) -> (w572:dbl[])
                        n442 = Build Array (concatenate)(w587, w588, w589, w590, w591, w592, w593, w586) -> (w569:dbl[])
                        n443 = local read "FF_Off_Ref"() -> (w574:refnum<file>)
                        n444 = local read "NF_Off_Ref"() -> (w571:refnum<file>)
                        n445 = local read "FF_Off_Ptr"() -> (w573:i64)
                        n446 = local read "NF_Off_Ptr"() -> (w570:i64)
                        n447 = Set File Position(offset (in bytes) (0)=w573, refnum=w574) -> (refnum out=w585:refnum<file>, error out=w583:errorcluster)  [unwired: 2 in]
                        n448 = Set File Position(offset (in bytes) (0)=w570, refnum=w571) -> (refnum out=w581:refnum<file>, error out=w579:errorcluster)  [unwired: 2 in]
                        n449 = Write to Binary File(file (use dialog)=w585, data=w572, error in=w583, 5:FALSE ("prepend array or string size? (T)")) -> (refnum out=w584:refnum<file>, error out=w582:errorcluster)  [unwired: 2 in, 1 out]
                        n450 = Write to Binary File(file (use dialog)=w581, data=w569, error in=w579, 5:FALSE ("prepend array or string size? (T)")) -> (refnum out=w580:refnum<file>, error out=w578:errorcluster)  [unwired: 2 in, 1 out]
                        n451 = Get File Position(4:w582, 7:w584) -> (2:w575:i64)  [unwired: 2 out]
                        n452 = Get File Position(4:w578, 7:w580) -> (2:w568:i64)  [unwired: 2 out]
                        n453 = local write "FF_Off_Ptr"(w575) -> ()
                        n454 = local write "NF_Off_Ptr"(w568) -> ()
                      }
                    }
                  }
                }
              }
              frame #4 {
                n455 = First Call?() -> (First Call?: T/F=w597:bool)
                n456 = Or(x="calculate absorption cross sections", y=w597) -> (x .or. y?=w595:bool)
                n457 = case shown="True" w595 {
                  frame False {
                  }
                  frame True {
                    # "calculate absorption cross sections from HITRAN data base"
                    n458 = local read "Off-Line Smoothed"() -> (w598:dbl[])
                    n459 = local read "Lambda On Read (nm)"() -> (w601:dbl)
                    n460 = local read "Lambda Off Set (nm)"() -> (w604:dbl)
                    n461 = local read "Temperature (C)"() -> (w602:dbl)
                    n462 = local read "Pressure (mb)"() -> (w603:dbl)
                    n463 = script code="%Importing HITRAN data\n%hitran = dlmread('C:\\Users\\H2ODial\\Desktop\\Shared Telescope WV DIAL Code\\Libraries and VIs\\824nm_841nm_H2O.csv', ',',[0 1 352 7]);\nhitran = dlmread('C:\\Users\\H2ODial\\Desktop\\Shared Telescope WV DIAL Code\\Libraries and VIs\\824nm_841nm_H2O_Spectral_Calc.csv', ',',[1 1 1209 7]);\n\n%Range vector in meters\nrange = ([75:75:size(Online,2)*75]);\n\nif lambda< 828\nlambda=828.195;\nelse\nlambda=lambda;\nend;\n\n%%\n\n%Voigt profile calculation\nWNmin = 12070.0;\nWNmax = 12076.0;\n\n%Find lines from WNmin to WNmax to calculate voigt profile\nline_indices = find(hitran(1:size(hitran,1),1)>WNmin & hitran(1:size(hitran,1),1)<WNmax);\n\nline = (hitran(line_indices, 1:size(hitran,2)));\n\n%Calculate temperature and pressure profile\nT0 = 273+15.6;\nT0 = 273+T0_C;\n\nT = T0-0.005545.*range; \n\nP0  = 1.0;\nP0  = P0_mb/1000*0.986; %pressure in mb converted to atm\n\nP = P0.*(T0./T).^-5.21986;\n\n%linewidth temperature dependence factor\nalpha = line(:,7);        \n\n%initial Lorentz linewidth from HiTRAN [cm^-1]\ngammal0 = line(:,4);     \n\n%ground state transition energy [cm^-1]\nE = line(:,6);           \n\n%initial linestrength from HiTRAN [cm^-1/(mol*cm^-2)]\nS0 = line(:,2);      \n\n%absorption line center wavenumber from HiTRAN [cm^-1]\nnu0_0 = line(:,1);    \n\nnu_on = (1/(lambda)*1e7);\n\nnu_off = (1/(lambda_off)*1e7);\n\n\nfor i = 1:size(Online,2);\n\n    %Pressure shift\n    nu0 = nu0_0-.0428.*P(i);\n    \n    %Calculate Lorentz lineweidth at temperature T [cm^-1]\n    gammal = gammal0.*(P(i)./P0).*((T0./T(i)).^alpha);\n    \n    %Calculate Doppler linewidth at temperature T [cm^-1]\n    gammad = (nu0).*((2.0.*1.38E-23.*T(i).*log(2.0))./(0.018.*3.0E8.*3.0E8./6.022E23)).^(0.5);\n    \n    y = (gammal./gammad).*((log(2.0)).^(0.5));\n    \n    x_on = ((nu_on-nu0)./gammad).*(log(2.0)).^(0.5);\n    \n    x_off = ((nu_off-nu0)./gammad).*(log(2.0)).^(0.5);\n    \n    %setting up Voigt convolution\n    stepsize = 1;\n    \n    t = [-200:1:199].*stepsize;\n    \n    t = repmat(t',1,length(x_on))';\n    \n    x_on = repmat(x_on,1,length(t));\n    \n    x_off = repmat(x_off,1,length(t));\n    \n    y = repmat(y,1,length(t));\n    \n    f_on = (exp(-t.^2.0))./(y.^2.0+(x_on-t).^2.0);\n    \n    f_off = (exp(-t.^2.0))./(y.^2.0+(x_off-t).^2.0);\n    \n    %Set the integration sum to zero to start\n    integral_on = 0.0;\n    \n    integral_off = 0.0;\n    \n    %Voigt integration\n    z_on = trapz(t(1,:),f_on,2);\n    \n    z_off =  trapz(t(1,:),f_off,2);\n    \n    integral_on = z_on;\n    \n    integral_off = z_off;\n    \n    %Calculate linestrength at temperature T\n    S = S0.*((T0./T(i)).^(1.5)).*exp(1.439.*E.*((1./T0)-(1./T(i))));\n    \n    %Calculate Doppler line-center cross section [cm^2]\n    K = (S./gammad).*(((log(2.0))./pi).^(0.5));\n    \n    %Calculate the Voigt profile\n    V_on = (y(1)/pi).*integral_on;\n    \n    V_off = (y(1)./pi).*integral_off;\n    \n    %Calculate the Voigt profile absorption cross section [cm^2]\n    sigmav_on = K.*V_on;\n    \n    sigmav_off = K.*V_off;\n    \n    %Sum contributions from all of the surrounding lines\n    sigma_on_total(i) = sum(sigmav_on);\n    \n    sigma_off_total(i) = sum(sigmav_off);\n    \nend;"("lambda"=w601, "lambda_off"=w604, "P0_mb"=w603, "T0_C"=w602, "Online"=w598) -> ("sigma_on_total"=→"sigma_on_total":dbl[], "sigma_off_total"=→"sigma_off_total":dbl[])  [unwired: 1 in, 1 out]
                  }
                }
              }
              frame #5 {
                w615 = 1
                # "normalization factor\nfrom 300 to 450m"
                # "OPTICAL DEPTH PLOT"
                # "new rainbow color bar display"
                # "Data Processing Far Channel"
                # "new rainbow color bar display"
                # "Calculating the range resolved water vapor number density and plotting"
                n464 = local read "sigma_off_total"() -> (w638:dbl[])
                n465 = local read "sigma_on_total"() -> (w635:dbl[])
                n466 = local read "On-Line  Smoothed"() -> (w613:dbl[])
                n467 = local read "Off-Line Smoothed"() -> (w612:dbl[])
                n468 = local read "Off-Line Smoothed 2"() -> (w636:dbl[])
                n469 = local read "On-Line Smoothed 2"() -> (w637:dbl[])
                n470 = script code="%Time averaging in seconds.  600 Seconds =10 minutes\ntemporal_average = 600;\n\n%Spatial averaging in bins.  2 bins = 150 meters\nspatial_average = 2;\n\n%Creating r and r+deltar vectors..this can also be acsomplished using the\n%diff command\np_oni = Online(:,1:size(Online,2)-1);\n\np_onii = Online(:,2:size(Online,2));\n\np_offi = Offline(:,1:size(Offline,2)-1);\n\np_offii = Offline(:,2:size(Offline,2));\n\nInside = (p_oni.*p_offii)./(p_onii.*p_offi);\n\ndel_cross = 1./(2.*(sigma_on_total(1:size(Online,2)-1)-sigma_off_total(1:size(Offline,2)-1)).*75*100);\n\ndel_cross(isinf(del_cross)) = 0;\n\n%Calculating Number density\nN = del_cross.*log(Inside);\n\n%Spatial smoothing of the profiles\nfilter1 = ones(1,2)./2;\n\nN_1 = N;\n\nN_1_avg = filter2(filter1,N_1);\n\nfilter1 = ones(1,10)./10;\n\nN_2 = N;\n\nN_2_avg = filter2(filter1,N_2);\n\nN_new = zeros(size(N,1),size(N,2));\n \n%Using different averaging windows for different altitudes \nN_avg=[N_1_avg(:,1:40)';N_2_avg(:,41:size(N,2))']';\n\n\nw = N_avg.*1e6.*18.015./6.022e23"("Online"=w637, "Offline"=w636, "sigma_on_total"=w635, "sigma_off_total"=w638) -> ("N_avg"=w639:cdb[], "w"=w648:cdb[])  [unwired: 1 in, 1 out]
                n471 = script code="%Time averaging in seconds.  600 Seconds = 10 minutes\ntemporal_average = 600;\n\n%Spatial averaging in bins.  2 bins = 150 meters\nspatial_average = 2;\n\n%Creating r and r+deltar vectors..this can also be acsomplished using the\n%diff command\np_oni = Online(:,1:size(Online,2)-1);\n\np_onii = Online(:,2:size(Online,2));\n\np_offi = Offline(:,1:size(Offline,2)-1);\n\np_offii = Offline(:,2:size(Offline,2));\n\nInside = (p_oni.*p_offii)./(p_onii.*p_offi);\n\ndel_cross = 1./(2.*(sigma_on_total(1:size(Online,2)-1)-sigma_off_total(1:size(Offline,2)-1)).*75*100);\n\ndel_cross(isinf(del_cross)) = 0;\n\n%Calculating Number density\nN = del_cross.*log(Inside);\n\n%Spatial smoothing of the profiles\nfilter1 = ones(1,2)./2;\n\nN_1 = N;\n\nN_1_avg = filter2(filter1,N_1);\n\nfilter1 = ones(1,10)./10;\n\nN_2 = N;\n\nN_2_avg = filter2(filter1,N_2);\n\nN_new = zeros(size(N,1),size(N,2));\n \n%Using different averaging windows for different altitudes \nN_avg=[N_1_avg(:,1:40)';N_2_avg(:,41:size(N,2))']';\n\n \nw = N_avg.*1e6.*18.015./6.022e23"("Online"=w613, "Offline"=w612, "sigma_on_total"=w635, "sigma_off_total"=w638) -> ("N_avg"=w644:cdb[], "w"=w645:cdb[])  [unwired: 1 in, 1 out]
                n472 = local read "Time Resolution Per Bin(ns)"() -> (w614:u32)
                n473 = local read "bins"() -> (w640:u32)
                n474 = local read "Altitude Array (km)"() -> (w610:dbl[])
                n475 = Build Array(w645, w648) -> (w651:cdb[][])
                n476 = To Double Precision Float(number=w614) -> (double precision float=w633:dbl)
                n477 = Reshape Array(w644, w615, w640) -> (w655:cdb[][])
                n478 = Reshape Array(w639, w615, w640) -> (w642:cdb[][])
                n479 = Multiply(x=0.15, y=w633) -> (x*y=w631:dbl)
                n480 = Build Array(w644, w639) -> (w649:cdb[][])
                n481 = Divide(x=300.0, y=w631) -> (x/y=w628:dbl)
                n482 = Divide(x=450.0, y=w631) -> (x/y=w627:dbl)
                n483 = Build Array(w610, w610) -> (w634:dbl[][])
                n484 = call "Convert to Dynamic Data5"("2D Array"=w651) -> ("Dynamic Data Type"=w650:dynamicdata)  [unwired: 3 in]
                n485 = call "Convert to Dynamic Data2"("2D Array"=w649) -> ("Dynamic Data Type"=w646:dynamicdata)  [unwired: 3 in]
                n486 = Divide(x=w655, y=1e+17) -> (x/y=→"Water Vapor Number Density":cdb[][])
                n487 = Divide(x=w642, y=1e+17) -> (x/y=→"Water Vapor Number Density 2":cdb[][])
                n488 = call "Convert to Dynamic Data6"("Array"=w610) -> ("Dynamic Data Type"=w611:dynamicdata)  [unwired: 3 in]
                n489 = To Long Integer(number=w628) -> (32bit integer=w626:i32)
                n490 = To Long Integer(number=w627) -> (32bit integer=w625:i32)
                n491 = call "Convert to Dynamic Data"("2D Array"=w634) -> ("Dynamic Data Type"=w647:dynamicdata)  [unwired: 3 in]
                n492 = call "Convert to Dynamic Data8"("2D Array"=w634) -> ("Dynamic Data Type"=w652:dynamicdata)  [unwired: 3 in]
                n493 = Decrement(x=w626) -> (x-1=w623:i32)
                n494 = Decrement(x=w625) -> (x-1=w624:i32)
                n495 = call "Build XY Graph"("Y Input"=w647, "X Input"=w646) -> ("XY Graph"=→"Water Vapor Number Density  2":cluster{"Y":dbl[], "Y":dbl[]}[])  [unwired: 3 in, 6 out]
                n496 = call "Build XY Graph3"("Y Input"=w652, "X Input"=w650) -> ("XY Graph"=→"Absolute Humidity":cluster{"Y":dbl[], "Y":dbl[]}[])  [unwired: 3 in, 6 out]
                n497 = Array Subset(array=w613, index=w623, length=w624) -> (w622:dbl[])
                n498 = Array Subset(array=w612, index=w623, length=w624) -> (w621:dbl[])
                n499 = call-poly <vilib>:"Mean.vi"("X"=w622) -> ("mean"=w620:dbl)  [unwired: 1 out]
                n500 = call-poly <vilib>:"Mean.vi"("X"=w621) -> ("mean"=w619:dbl)  [unwired: 1 out]
                n501 = Divide(x=w620, y=w619) -> (x/y=w618:dbl)
                n502 = Multiply(x=w612, y=w618) -> (x*y=w617:dbl[])
                n503 = Divide(x=w613, y=w617) -> (x/y=w616:dbl[])
                n504 = Natural Logarithm(1:w616) -> (0:w607:dbl[])
                n505 = Multiply(x=-1.0, y=w607) -> (x*y=w606:dbl[])
                n506 = call "Convert to Dynamic Data9"("Array"=w606) -> ("Dynamic Data Type"=w609:dynamicdata)  [unwired: 3 in]
                n507 = call "Build OD Plot"("Y Input"=w611, "X Input"=w609) -> ("XY Graph"=→"Optical Depth":cluster{"Y":dbl[], "Y":dbl[]}[])  [unwired: 3 in, 6 out]
              }
            }
          }
        }
        "L_Count" <- w126
      }
    }
  }
  n508 = case shown="True" w3 {
    frame False {
    }
    frame True {
      # "close data files"
      n509 = local read "NF_Off_Ref"() -> (w658:refnum<file>)
      n510 = local read "NF_On_Ref"() -> (w659:refnum<file>)
      n511 = local read "FF_Off_Ref"() -> (w660:refnum<file>)
      n512 = local read "FF_On_Ref"() -> (w661:refnum<file>)
      n513 = Close File(refnum=w661) -> ()  [unwired: 1 in, 2 out]
      n514 = Close File(refnum=w660) -> ()  [unwired: 1 in, 2 out]
      n515 = Close File(refnum=w659) -> ()  [unwired: 1 in, 2 out]
      n516 = Close File(refnum=w658) -> ()  [unwired: 1 in, 2 out]
    }
  }
  "FileHour" <- -1 ("FileHour")
  "DataOpen" <- FALSE
